vi "SEC code V4.9.vi"() -> ()   [LabVIEW 2022 SP3]
uses:
  SEC code V3.1/Drivers and Aux files/user.lib/atmcd32d.llb/Shutter_type typedef.ctl
  C:/SEC Software V4.91/EcoChemie.Autolab.Sdk.dll
  EcoChemie.Autolab.Sdk.dll
  SEC code V3.1/Drivers and Aux files/State.ctl
  SEC code V3.1/Drivers and Aux files/SECenumctl.ctl
  SEC code V3.1/Drivers and Aux files/user.lib/atmcd32d.llb/TriggerMode_mode typedef.ctl
  SEC code V3.1/Drivers and Aux files/OSSPEC.ctl
  SEC code V3.1/Drivers and Aux files/OSPEC-enum.ctl
  Labview/IVIUM/IVIUM_remdriver.lvlib
panel:
  out "Current PD 2":dbl
  out "POtential PD 2":dbl
  in  "Tab Control 5":enum32{"AUTOLAB", "IVIUM", "iDUS", "Kymera"}(tab)
  out "current":dbl
  out "Error after autolab connection?":errorcluster
  out "Autolab Connected?":bool
  out "Voltage":dbl format="%#_3e"
  out "PotentialOverload":bool
  out "Bandwidth":i32
  out "CurrentRange":i32
  out "Mode":i32
  out "Measured voltage":dbl
  out "CurrentOverload":bool
  out "Cell on?":bool
  out "current":dbl caption="Current (A)" format="%_4g"
  out "cell on":bool
  out "V (during measurment)":dbl
  out "Potentiostat Status":string
  out "T reached?":bool
  out "Shut down sequence run?":bool
  out "Curent Temp":i32
  in  "Tab Control 4":T1(tab)
  in  "Use autolab?":bool=TRUE
  in  "Embedded Exe File":path=path "C:/Program Files/Metrohm Autolab/Autolab SDK 2.1/Hardware Setup Files/Adk.x"
  in  "Hardware Setup File":path=path "C:/ProgramData/Metrohm Autolab/13.0/HardwareSetup.AUT55157.xml"
  in  "Bandwidth 2":i32(ring)=2 items=["UltraHigh_Speed", "High_Speed", "High_Stability"]
  in  "Start potential (V)":dbl=0.2
  in  "Stop potential (V)":dbl=0.7
  in  "Increment (V)":dbl=0.05
  in  "Default Potential (V)":dbl=0.2
  in  "Wait before \nspectrum (s)":dbl=0.1
  in  "Equilibration \ntime (s)":u32=5
  in  "Reverse Scan\ndirection":bool
  in  "(update and read)":bool
  in  "Tab Control 3":T2(tab)=enum."iDUS run"
  in  "Inetegration\n Time (us)":i32=5000
  in  "Continuous \nStrobe Delay (us)":i32
  in  "Number of averages":i32
  in  "Use iDus?":bool=TRUE
  in  "Return detector \nto room T?":bool
  in  "Init, Cool, read dark,\nOR\nWarm/de-init detector":bool
  in  "Temperature\n(degrees C)":i32=-80
  in  "Number of scans in kinetic cycle":i32=30
  in  "Exposure time (s)":dbl=0.03
  in  "Tab Control 2":T3(tab)
  in  "V 1 time (s)":dbl=10.0
  in  "V off time":dbl=30.0
  in  "Sampling\n delay (s)":dbl
  in  "V 2 time (s)":dbl=20.0
  in  "Run OSPSEC":bool
  in  "Square wave?":bool
  out "OCP I (close to 0)":dbl
  out "OCP":dbl format="%_3f"
  in  "V1 (V)":dbl=0.4
  in  "V2 (V)":dbl=0.8
  in  "Slow sample time (s)":dbl=1500.0
  out "Time during PD":u32
  in  "File Name":string="test-1"
  in  "File Path":path=path "C:/Data"
  in  "Tab Control":T4(tab)
  out "?":T5(graph)
  out "?":cluster{i32[], dbl[]}(graph)
  out "?":T5(graph)
  out "?":T5(graph)
  out "Current during PD":dbl(graph)=1.602783203125e-06
  out "?":cluster{dbl[], dbl[]}(graph)
  out "Potential  During PD":dbl(graph)=-0.0002471923828124972
  out "Setpoint":dbl
  out "?":cluster{i32[], "array":i32[]}(graph)
  out "I_overload":bool
  out "Aninput1_overload":bool
  out "E_overload":bool
  out "cell-off button pressed":bool
  in  "Default\nCurrent range":T6(ring)=enum."100 uA"
  in  "Default Filter":T7(ring)=enum."10 kHz"
  out "Device serial number":string
  in  "Set Stability":T8(ring)=enum."Standard"
  out "Number of Spectrometers":i32
  out "IDus not in read loop? (kinetic)":bool
  out "Get status return code":dbl
  out "xpixels":i32
  out "ypixels":i32
  out "Calculated exposure time":sgl format="%.2f"
  out "Check timings return code":u32
  out "Set temprature\nreturn code":u32
  out "get aquired data return code":u32
  out "Start Aquisition return code":u32
  out "Init. return code":u32
  out "Cooler Off return code":u32
  out "Time before the start of current aquisition (ms)":u32
  out "Time  after the aquisition (before fetch data), (ms)":u32
  in  "Shutter opens on TTL":T9=enum."TTL High"
  in  "Shutter open and close time":i32
  out "Get aqisition ok? (kinetic mode)":bool
  out "Time taken to apply V2":u32
  out "Values to re-intialise to at end\nof the measument":T10
  out "V2 applied?":bool
  out "ContinuousStrobe Out":u32
  out "Wrapper Out":u32
  out "WL Values":dbl[](array[numeric])
  out "Number of time the OCEAN averaging loop has run -1":i32
  out "Adc":refnum<k24>
  out "Sampler 2":refnum<k24>
  out "Dio":refnum<k24>
  out "Dac":refnum<k24>
  out "instrument":refnum<k24>
  out "Ei":refnum<k24>
  out "AutolabConnection":refnum<k24>
  out "EI status supported for":string[](array[string])
  out "TemperatureOverload":bool
  out "ManualCellSwitch":bool
  out "Oscillation":bool
  out "PD ENDED\nEXIT MEASURMENT":bool=TRUE
  out "Current PD":dbl
  out "POtential PD":dbl
  in  "Exit and disconnect":bool
  # "Program control"
  # "Potential decay control"
  # "Spectrometer control"
  # "System status"
  # "SEC control"
  # "Cell on?"
  # "Use the integration time program in the same folder as this program\nto get the optimum value. For kinetic mode the time resolution is limited \nby integration time"
  # "Unless you know what you are doing keep these at 0.03 and 30"
  # "I overload overload"
  # "off button pressed"
  # "Aninput1 overload"
  # "E overload"
  # "OSPEC loop exit"
  # "Checklist for avoiding errors:\n(1) Light on the IVIUM should be blue with red flashes\nIf the system crahes and the light is red then connect and disconnect in IVUM soft/turn stat off/on\n(2) Maya Pro should read in ocean view/or the get intensity program\nIf maya is not reading connect and disconnect USB.\n(3) If errors persist rrepeat steps 1 + 2 then re-compile code by clicking the\nwhite (run) whilst holding down CRTL + (left) SHIFT\n(4) IF USING THE iDus DO NOT EXIT WITHOUT WARMING CAMERA BACK TO ROOM T,YOU \nWILL DAMAGE IT \n(6) if the IVIUM.dll does not load click broken arrows and \"show error\" until you see the call library function (see blue circles). Double click on this and paste the following into the directory (red circle):   \n%windir%\\Labview\\IVIUM\\IVIUM_remdriver.dll"
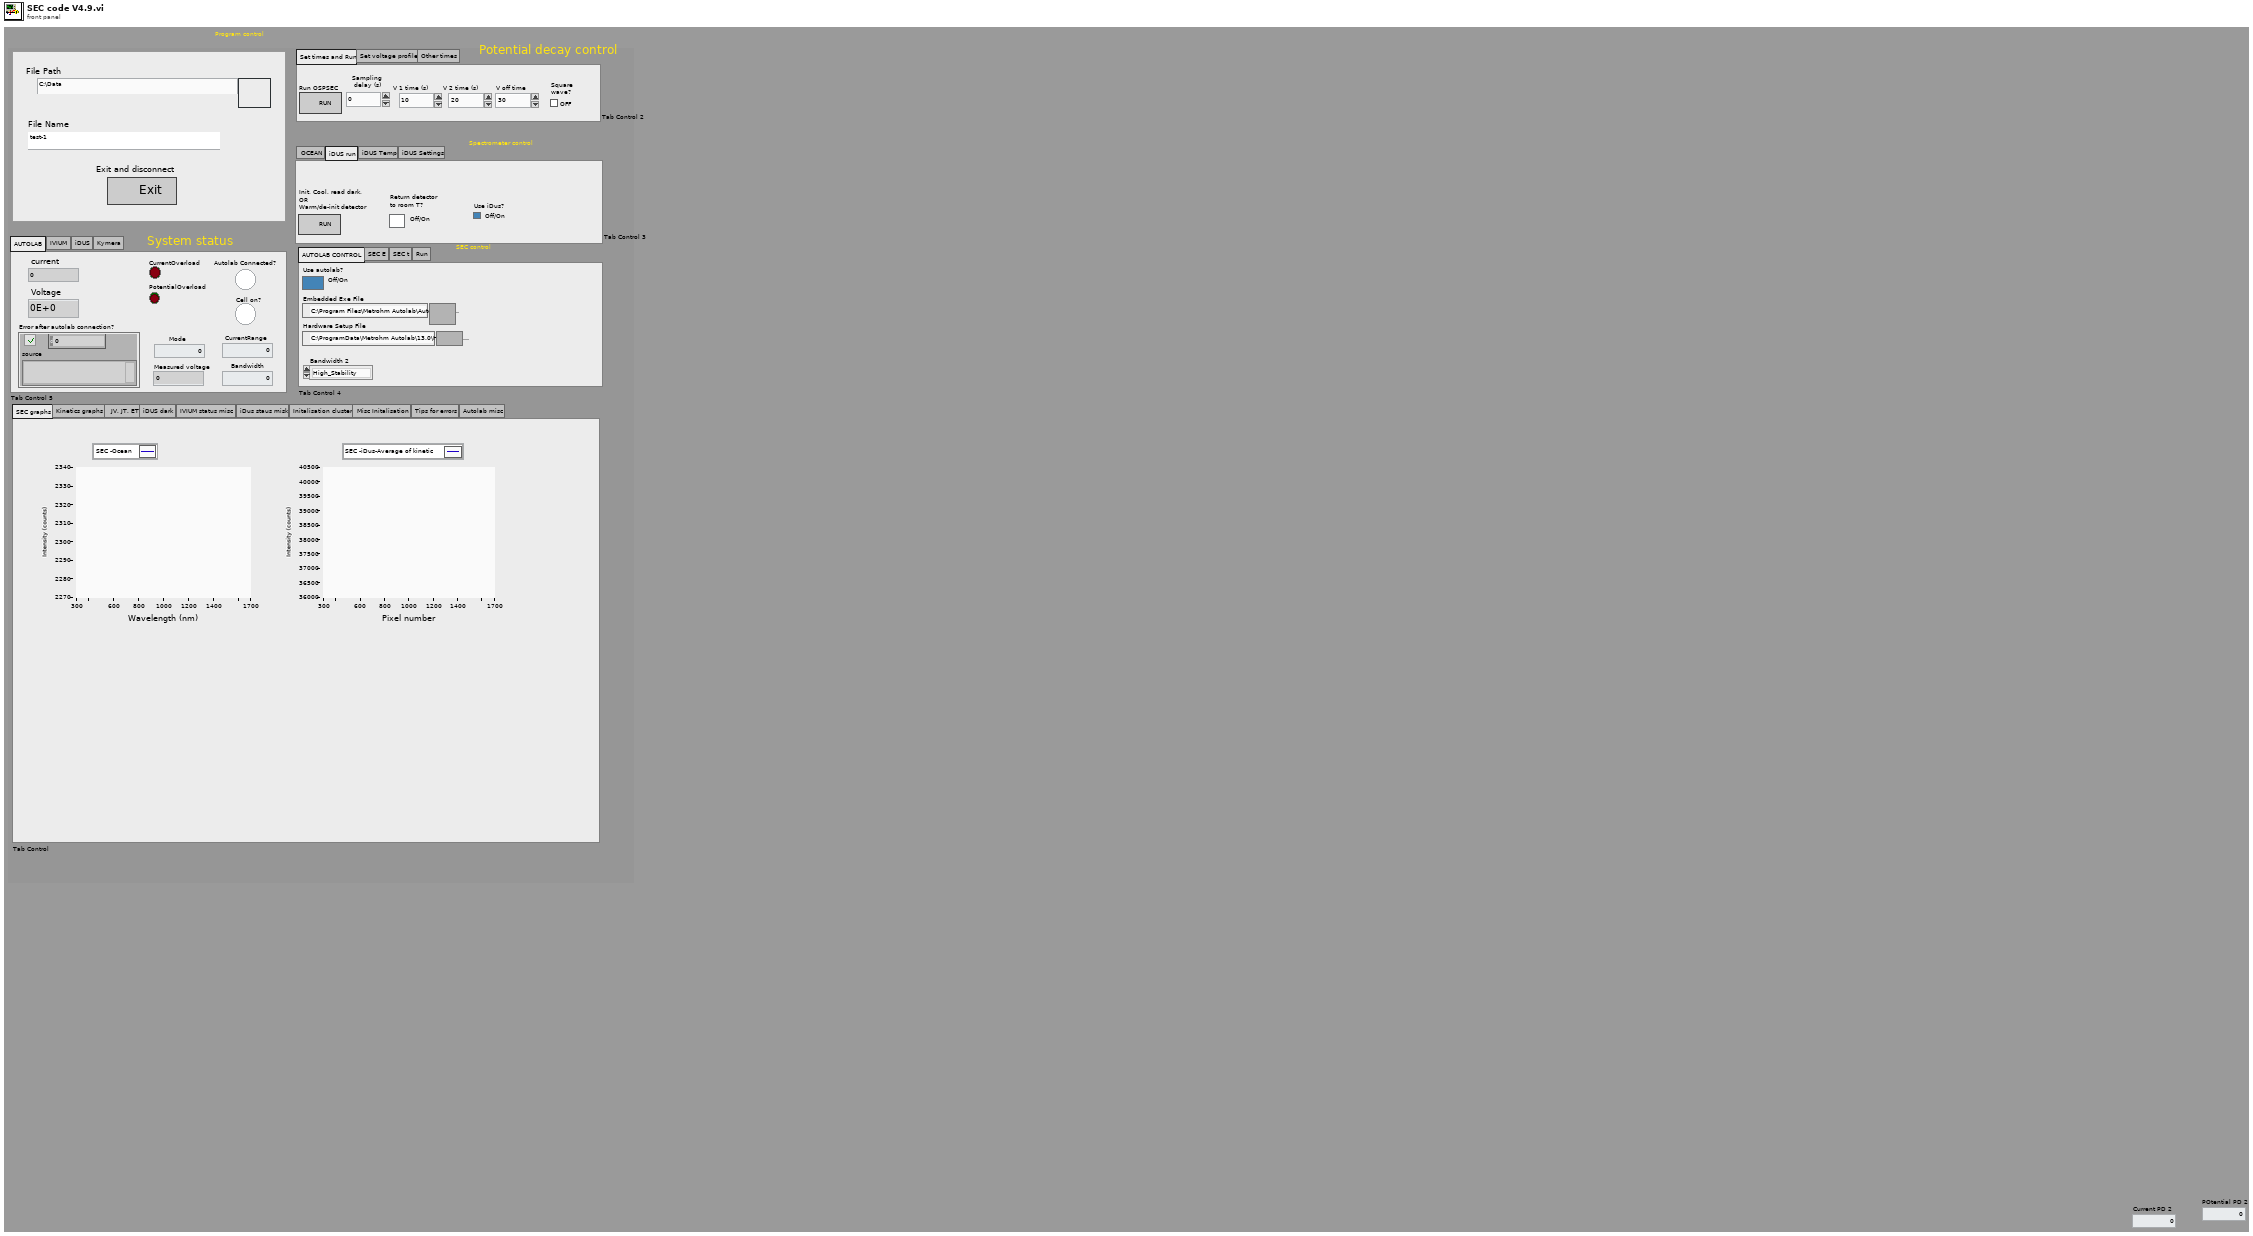
[diagram p1: front panel]
types:
  T1 = enum32{"AUTOLAB CONTROL", "SEC E", "SEC t", "Run"}
  T2 = enum32{"OCEAN", "iDUS run", "iDUS Temp", "iDUS Settings"}
  T3 = enum32{"Set times and Run", "Set voltage profile", "Other times"}
  T4 = enum32{"SEC graphs", "Kinetics graphs", " JV, JT, ET", "iDUS dark", "IVIUM status misc", "iDus staus misk", "Initalisation cluster", "Misc Initalisation ", "Tips for errors", "Autolab misc"}
  T5 = cluster{"WL Values":dbl[], "Spectrum Values":dbl[]}
  T6 = enum16{"10 A", "1 A", "100 mA", "10 mA", "1 mA", "100 uA", "10 uA", "1 uA", "100 nA", "10 nA", "1 nA", "100 pA", "10 pA", "1 pA"}
  T7 = enum16{"1 MHz", "100 kHz", "10 kHz", "1 kHz", "10 Hz"}
  T8 = enum16{"High Speed", "Standard", "High Stability"}
  T9 = typedef "Shutter_type typedef.ctl" = enum16{"TTL Low", "TTL High"}
  T10 = cluster{"Currents":dbl[], "Potentials":dbl[], "Device Status":string, "Device serial no":string, "Current":dbl, "Default \nPotential":dbl, "I overload":bool, "Cell On":bool, "E overload":bool, "Aninput1 overload":bool, "Cell off button pressed":bool, "Start potential":dbl, "Stop potential":dbl, "Increment":dbl, "SEC":dbl[], "Path":path, "File name":string}
  T11 = cluster{"Current array":dbl[], "Potential array":dbl[], "Status":string, "Serial No":string, "Current":dbl, "Default\n potential":dbl, "I overload":bool, "Cell on":bool, "E overload":bool, "Cell of button pressed":bool, "Aninput1 overload":bool, "Stop \npotential":dbl, "Start \npotential":dbl, "Increment":dbl, "Spectrum":dbl[][], "Path":path, "File Name":string, "Sample rate":dbl, "V2 time":dbl, "V off time":dbl, "V 2":dbl, "V 1":dbl, "V1 time":dbl, "Time array":dbl[], "Integration time":i32, "Continous strobe delay":i32, "Time elapsed ":i32, "Start time":i32, "Time for E measurment":i32[], "Time for I measurment ":i32[], "Time for spectrum measurment":i32[], "Return detector to \nroom T":bool, "Number of scans in kinetic cycle":i32, "Exposure time":dbl}
  T12 = typedef "State.ctl" = enum16{"Initialize", "Wait for Event", "Run SEC", "Run OSPEC", "Initialse and cool iDus", "Exit"}
  T13 = typedef "SECenumctl.ctl" = enum16{"Read spectrum from Ocean", "Read spectrum from iDus", "Apply potential", "Wait", "Apply potential Autolab"}
  T14 = typedef "TriggerMode_mode typedef.ctl" = enum16{"Internal", "External", "N/A (2)", "N/A (3)", "N/A (4)", "N/A (5)", "External Start", "External Exposure (Bulb)", "N/A (8)", "External FVB EM", "Software", "N/A (11)", "External Charge Shifting"}
  T15 = typedef "OSSPEC.ctl" = enum16{"Read Potential and spectrum", "Read current and spectrum", "Reinitialise Cell", "Apply V1", "End measurment", "Apply V2"}
  T16 = typedef "OSPEC-enum.ctl" = enum16{"Check exit", "Read", "Wait"}
  T17 = enum16{"off", "EStat4EL", "EStat2EL", "EStatDummy1", "EStatDummy2", "EStatDummy3", "EStatDummy4", "IStat4EL", "IStat2EL", "IStatDummy", "BiStat4EL", "BiStat2EL"}
  T18 = cluster{"Current array":dbl[], "Potential array":dbl[], "Status":string, "Serial No":string, "Current":dbl, "Default\n potential":dbl, "I overload":bool, "Cell on":bool, "E overload":bool, "Cell of button pressed":bool, "Aninput1 overload":bool, "Stop \npotential":dbl, "Start \npotential":dbl, "Increment":dbl, "Spectrum":dbl[][], "Path":path, "File Name":string, "Sample rate":dbl, "V2 time":dbl, "V off time":dbl, "V 2":dbl, "V 1":dbl, "V1 time":dbl, "Time array":dbl[], "Integration time":i32, "Continous strobe delay":i32, "Time elapsed ":i32, "Start time":i32, "Time for E measurment":i32[], "Time for I measurment ":i32[], "Time for spectrum measurment":i32[], "Return detector to \nroom T":bool, "Number of scans in kinetic cycle":i32, "Exposure time":i32}
  T19 = typedef "Error Code Enum typedef.ctl" = enum32{"N/A (0)", "DRV_ERROR_CODES", "DRV_SUCCESS", "DRV_VXDNOTINSTALLED", "DRV_ERROR_SCAN", "DRV_ERROR_CHECK_SUM", "DRV_ERROR_FILELOAD", "DRV_UNKNOWN_FUNC", "DRV_ERROR_VXD_INIT", "DRV_ERROR_ADDRESS", "DRV_ERROR_PAGELOCK", "DRV_ERROR_PAGEUNLOCK", "DRV_ERROR_BOARDTEST", "DRV_ERROR_ACK", "DRV_ERROR_UP_FIFO", "DRV_ERROR_PATTERN", "N/A (16)", "DRV_ACQUISITION_ERRORS", "DRV_ACQ_BUFFER", "DRV_ACQ_DOWNFIFO_FULL", "DRV_PROC_UNKONWN_INSTRUCTION", "DRV_ILLEGAL_OP_CODE", "DRV_KINETIC_TIME_NOT_MET", "DRV_ACCUM_TIME_NOT_MET", "DRV_NO_NEW_DATA", "N/A (25)", "DRV_SPOOLERROR", "N/A (27)", "N/A (28)", "N/A (29)", "N/A (30)", "N/A (31)", "N/A (32)", "DRV_TEMPERATURE_CODES", "DRV_TEMPERATURE_OFF", "DRV_TEMPERATURE_NOT_STABILIZED", "DRV_TEMPERATURE_STABILIZED", "DRV_TEMPERATURE_NOT_REACHED", "DRV_TEMPERATURE_OUT_RANGE", "DRV_TEMPERATURE_NOT_SUPPORTED", "DRV_TEMPERATURE_DRIFT", "N/A (41)", "N/A (42)", "N/A (43)", "N/A (44)", "N/A (45)", "N/A (46)", "N/A (47)", "N/A (48)", "DRV_GENERAL_ERRORS", "DRV_INVALID_AUX", "DRV_COF_NOTLOADED", "DRV_FPGAPROG", "DRV_FLEXERROR", "DRV_GPIBERROR", "N/A (55)", "N/A (56)", "N/A (57)", "N/A (58)", "N/A (59)", "N/A (60)", "N/A (61)", "N/A (62)", "N/A (63)", "DRV_DATATYPE", "DRV_DRIVER_ERRORS", "DRV_P1INVALID", "DRV_P2INVALID", "DRV_P3INVALID", "DRV_P4INVALID", "DRV_INIERROR", "DRV_COFERROR", "DRV_ACQUIRING", "DRV_IDLE", "DRV_TEMPCYCLE", "DRV_NOT_INITIALIZED", "DRV_P5INVALID", "DRV_P6INVALID", "DRV_INVALID_MODE", "DRV_INVALID_FILTER", "DRV_I2CERRORS", "DRV_I2CDEVNOTFOUND", "DRV_I2CTIMEOUT", "DRV_P7INVALID", "N/A (84)", "N/A (85)", "N/A (86)", "N/A (87)", "N/A (88)", "N/A (89)", "DRV_IOCERROR", "DRV_VRMVERSIONERROR"}
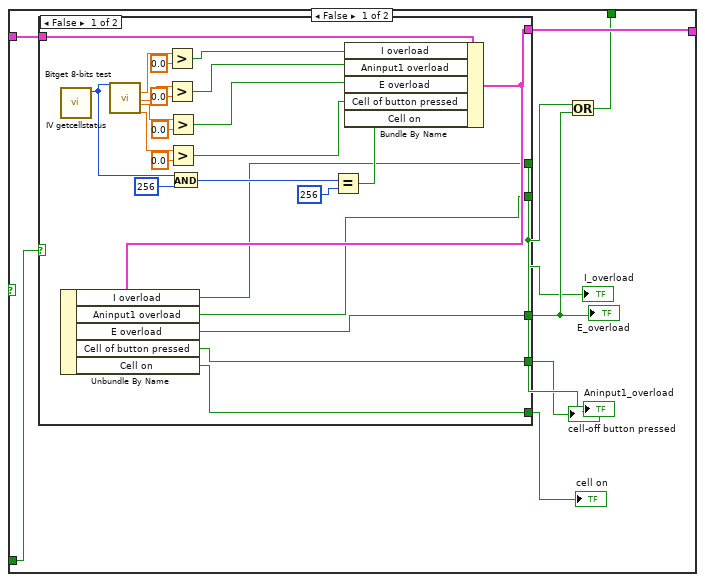
[diagram p2: hidden frame]
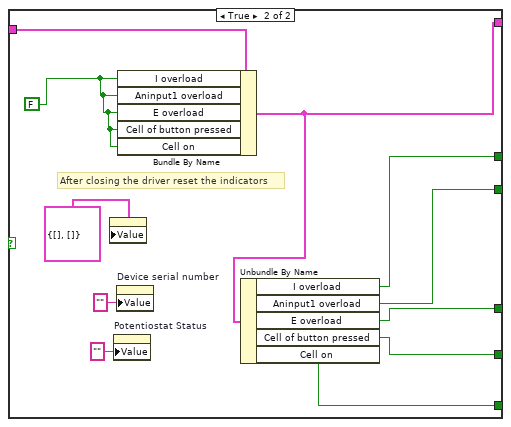
[diagram p3: hidden frame]
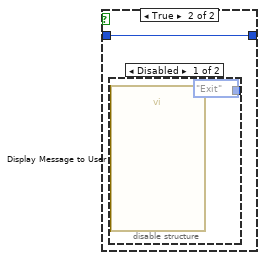
[diagram p4: hidden frame]
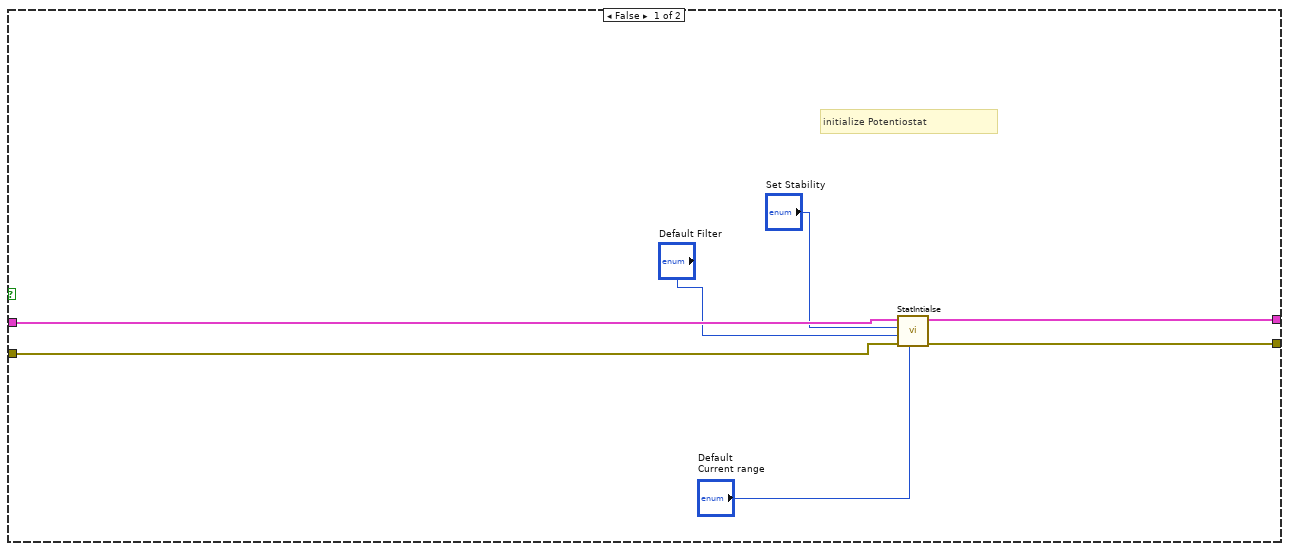
[diagram p7: hidden frame]
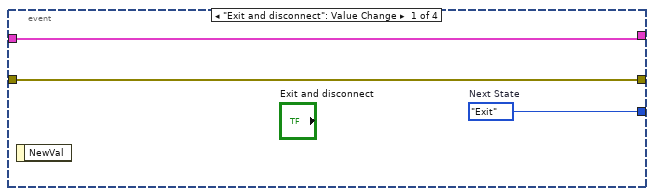
[diagram p9: hidden frame]
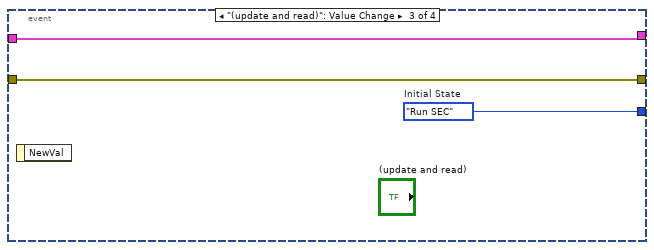
[diagram p10: hidden frame]
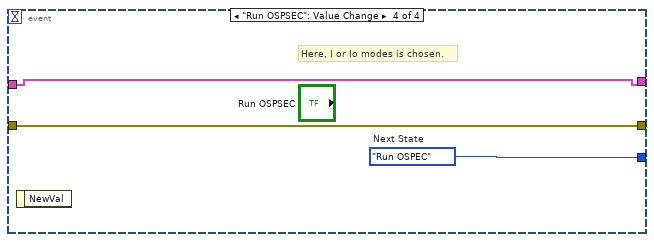
[diagram p11: hidden frame]
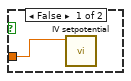
[diagram p12: hidden frame]
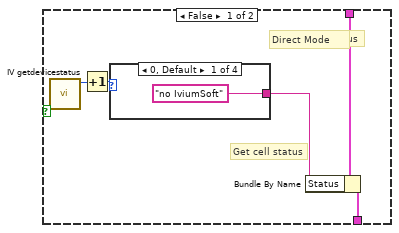
[diagram p13: hidden frame]
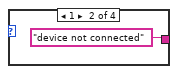
[diagram p14: hidden frame]
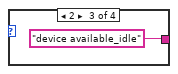
[diagram p15: hidden frame]
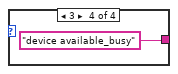
[diagram p16: hidden frame]
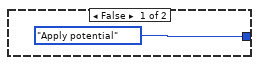
[diagram p17: hidden frame]
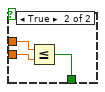
[diagram p20: hidden frame]
diagram:
  w1 = T11 {"Current array"=[], "Potential array"=[], "Status"="", "Serial No"="", "Current"=0.0, "Default\n potential"=0.0, "I overload"=FALSE, "Cell on"=FALSE, "E overload"=FALSE, "Cell of button pressed"=FALSE, "Aninput1 overload"=FALSE, "Stop \npotential"=0.0, "Start \npotential"=0.0, "Increment"=0.0, "Spectrum"=[], "Path"=path "", "File Name"="", "Sample rate"=0.0, "V2 time"=0.0, "V off time"=0.0, "V 2"=0.0, "V 1"=0.0, "V1 time"=0.0, "Time array"=[], "Integration time"=0, "Continous strobe delay"=0, "Time elapsed "=0, "Start time"=0, "Time for E measurment"=[], "Time for I measurment "=[], "Time for spectrum measurment"=[], "Return detector to \nroom T"=FALSE, "Number of scans in kinetic cycle"=0, "Exposure time"=0.0}  # Init cluster
  w3 = State."Initialize"  # Initial State
  n1 = while {
    shift-right: [w21] -> _
    shift-left: w3 -> [w38]
    shift-right: [w24] -> _
    shift-left: w1 -> [w17]
    shift-right: [w25] -> _
    shift-left: errorcluster {"status"=FALSE, "code"=0, "source"=""} ("error constant") -> [w37]
    stop <- w35 stop-if-true
    # "Main VI State Machine"
    n2 = Bundle By Name(cluster=w17, "Sample rate"="Sampling\n delay (s)", "V1 time"="V 1 time (s)", "V2 time"="V 2 time (s)", "V off time"="V off time", "V 2"="V2 (V)", "V 1"="V1 (V)", "Integration time"="Inetegration\n Time (us)", "Continous strobe delay"="Continuous \nStrobe Delay (us)", "Exposure time"="Exposure time (s)", "Number of scans in kinetic cycle"="Number of scans in kinetic cycle") -> (w11:T11)
    n3 = Bundle By Name(cluster=w11, "Default\n potential"="Default Potential (V)", "Start \npotential"="Start potential (V)", "Stop \npotential"="Stop potential (V)", "Increment"="Increment (V)", "Path"="File Path", "File Name"="File Name") -> (w23:T11)
    n4 = case shown="\"Run SEC\"" w38 {
      tunnel: [w94 w137 w185 w504 w544 w1716] -> w7
      tunnel: [w93 w134 FALSE ("Stop Loop?") w501 FALSE ("Stop Loop?") _] -> w36
      tunnel: w23 -> [w91 w131 w174 w505 w543 w1714]
      tunnel: [w90 w132 w159 w505 w539 w1714] -> w31
      tunnel: w37 -> [w95 w136 w183 w507 w541 w1713]
      tunnel: [w96 w135 w182 w508 w540 w1713] -> w25
      tunnel: [1 ("devconnect") 1 ("devconnect") 1 ("devconnect") w506 1 ("devconnect") 1 ("devconnect")] -> w22
      frame "Initialize" {
        w93 = FALSE  # Stop Loop?
        w94 = State."Wait for Event"  # Next State
        # "Initialize - Initialize variables needed"
        n5 = case shown="True" "Use autolab?" {
          tunnel: [w104 w109] -> w96
          tunnel: w95 -> [w103 _]
          tunnel: w91 -> [w102 w111]
          tunnel: [w98 w111] -> w90
          frame False {
            # "initialize Potentiostat"
            n6 = call "StatIntialse.vi"("Init cluster 2"=w102, "Set Stability"="Set Stability", "Default\n Filter"="Default Filter", "error in (no error)"=w103, "Default\nCurrent range"="Default\nCurrent range") -> ("Init cluster"=w98:T18, "error out"=w104:errorcluster)  [unwired: 4 in]
          }
          frame True {
            w108 = 2 items=["UltraHigh_Speed", "High_Speed", "High_Stability"] ("Bandwidth")
            w113 = 0 items=["Potentiostatic", "Galvanostatic"] ("Mode")
            w114 = -4 items=["CR07_1A"=0, "CR06_10A"=1, "CR01_100A"=2, "CR00_1000A"=3, "CR05_20A"=20, "CR04_40A"=40, "CR03_50A"=60, "CR02_80A"=80, "CR19_1pA"=-12, "CR18_10pA"=-11, "CR17_100pA"=-10, "CR16_1nA"=-9, "CR15_10nA"=-8, "CR14_100nA"=-7, "CR13_1uA"=-6, "CR12_10uA"=-5, "CR11_100uA"=-4, "CR10_1mA"=-3, "CR09_10mA"=-2, "CR08_100mA"=-1] ("CurrentRange")
            w115 = 1 items=["Off", "On"] ("CellOnOff")
            n7 = call "Connect AutoLab.vi"("Embedded Exe File"="Embedded Exe File", "Hardware Setup File"="Hardware Setup File") -> ("error out"=w120:errorcluster, ".NET Refnum out"=w129:refnum<k24>)  [unwired: 8 in]
            "Error after autolab connection?" <- w120
            n8 = property class="Instrument"(reference=w129, error in=w120) -> (reference out=→"instrument":refnum<k24>, error out=w121:errorcluster, "Adc"=→"Adc":refnum<k24>, "Dac"=→"Dac":refnum<k24>, "Dio"=→"Dio":refnum<k24>, "AutolabConnection"=w117:refnum<k24>, "Ei"=w107:refnum<k24>)
            "AutolabConnection" <- w117
            n9 = property class="AutolabConnection"(reference=w117) -> ("IsConnected"=→"Autolab Connected?":bool)  [unwired: 1 in, 2 out]
            n10 = property class="EI"(reference=w107, error in=w121) -> (reference out=→"Ei":refnum<k24>, error out=w128:errorcluster, "Sampler"=→"Sampler 2":refnum<k24>)
            n11 = Unbundle By Name(w111) -> ("Default\n potential"=w110:dbl)
            n12 = Build Array(w121, w128) -> (w122:errorcluster[])
            n13 = Merge Errors(w122) -> (w112:errorcluster)
            n14 = property class="EI" props=["Bandwidth", "CellOnOff", "CurrentRange", "Mode", "Setpoint", "Current", "Potential", "PotentialApplied", "PotentialOverload", "Sampler", "Setpoint", "PotentialOverload"](reference=w107, error in=w112, "Bandwidth"=w108, "CellOnOff"=w115, "CurrentRange"=w114, "Mode"=w113, "Setpoint"=w110) -> (error out=w109:errorcluster)  [unwired: 8 out]
            n15 = property class="EI"(reference=w107) -> ("Potential"=w106:dbl, "Current"=w105:dbl)  [unwired: 1 in, 2 out]
            n16 = property on="current" class="DigNum (strict)"("Value"=w105) -> ()  [unwired: 2 in, 2 out]
            n17 = property on="Voltage" class="DigNum (strict)"("Value"=w106) -> ()  [unwired: 2 in, 2 out]
          }
        }
        n18 = property on="V2 applied?" class="Bool (strict)"("Value"=FALSE ("V2 applied")) -> ()  [unwired: 2 in, 2 out]
        "Values to re-intialise to at end\nof the measument" <- T10 {"Currents"=[], "Potentials"=[], "Device Status"="", "Device serial no"="", "Current"=0.0, "Default \nPotential"=0.0, "I overload"=FALSE, "Cell On"=FALSE, "E overload"=FALSE, "Aninput1 overload"=FALSE, "Cell off button pressed"=FALSE, "Start potential"=0.0, "Stop potential"=0.0, "Increment"=0.0, "SEC"=[], "Path"=path "", "File name"=""} ("Values to re-intialise to at end\nof the measument")
      }
      frame "Wait for Event" {
        w134 = FALSE  # Stop Loop?
        # "Wait for Event - Use an Event Structure to monitor the user interface for events that run different states of the state machine."
        n19 = event shown="[1] \"Init, Cool, read dark, OR Warm/de-init detector\": Value Change" {
          selector: _ -> [_ _ _ _]
          dyn-events: _ -> [_ _ _ _]
          timeout: _ -> [_ _ _ _]
          tunnel: [w140 State."Initialse and cool iDus" ("Next State") w147 w151] -> w137
          tunnel: w136 -> [w139 w145 w148 w150]
          tunnel: [w139 w145 w148 w150] -> w135
          tunnel: w131 -> [w138 w143 w146 w149]
          tunnel: [w138 w141 w146 w149] -> w132
          event "Exit and disconnect": Value Change {
            w140 = State."Exit"  # Next State
            n20 = event-data() -> ()  [unwired: 1 in, 1 out]
          }
          event "Init, Cool, read dark,\nOR\nWarm/de-init detector": Value Change {
            n21 = event-data() -> ()  [unwired: 1 in, 4 out]
            n22 = Bundle By Name(cluster=w143, "Return detector to \nroom T"="Return detector \nto room T?") -> (w141:T11)
          }
          event "(update and read)": Value Change {
            w147 = State."Run SEC"  # Initial State
            n23 = event-data() -> ()  [unwired: 1 in, 1 out]
          }
          event "Run OSPSEC": Value Change {
            w151 = State."Run OSPEC"  # Next State
            # "Here, I or Io modes is chosen."
            n24 = event-data() -> ()  [unwired: 1 in, 1 out]
          }
        }
      }
      frame "Run SEC" {
        w185 = State."Wait for Event"  # Next State
        n25 = property on="Use autolab?" class="Bool (strict)"() -> ("Value"=w154:bool)  [unwired: 2 in, 2 out]
        n26 = case shown="True" w154 {
          tunnel: w174 -> [w191 w199]
          tunnel: [w190 w199] -> w161
          frame False {
            # "Get cell status"
            # "Get Device Status"
            # "Direct Mode"
            n27 = call "IV getdevicestatus.vi"() -> ("return type"=w193:i32)  [unwired: 10 in, 1 out]
            n28 = Increment(x=w193) -> (x+1=w192:i32)
            n29 = case shown="0, Default" w192 {
              tunnel: ["no IviumSoft" "device not connected" "device available_idle" "device available_busy"] -> w194
              frame 0, Default {
              }
              frame 1 {
              }
              frame 2 {
              }
              frame 3 {
              }
            }
            n30 = Bundle By Name(cluster=w191, "Status"=w194) -> (w190:T11)
          }
          frame True {
          }
        }
        n31 = property on="Use autolab?" class="Bool (strict)"() -> ("Value"=w156:bool)  [unwired: 2 in, 2 out]
        n32 = case shown="True" w156 {
          tunnel: [SECenumctl."Apply potential" SECenumctl."Apply potential Autolab"] -> w181
          frame False {
          }
          frame True {
          }
        }
        n33 = Unbundle By Name(w161) -> ("Increment"=w180:dbl, "Start \npotential"=w184:dbl, "Stop \npotential"=w175:dbl)
        n34 = while {
          shift-right: [w227] -> w158
          shift-left: w161 -> [w228]
          tunnel: w180 -> [w223]
          tunnel: w184 -> [w222]
          shift-right: [w224] -> w182
          shift-left: w183 -> [w225]
          shift-right: [w216] -> _
          shift-left: w181 -> [w220]
          shift-right: [w218] -> w160
          shift-left: dbl[] [0.0] -> [w217]
          shift-right: [w213] -> w164
          shift-left: dbl[] [0.0] -> [w214]
          tunnel: w175 -> [w215]
          shift-right: [w212] -> w173
          shift-left: dbl[][] [] -> [w211]
          tunnel: "Reverse Scan\ndirection" -> [w210]
          tunnel: [w208] -> _
          tunnel: [w208] -> _
          shift-right: [w207] -> _
          shift-left: -3 ("y") -> [w206]
          i -> [w226]
          stop <- w208 stop-if-true
          n35 = case shown="\"Apply potential Autolab\"" w220 {
            tunnel: w228 -> [w251 w315 w350 w365 w463]
            tunnel: [w250 w314 w350 w365 w463] -> w227
            tunnel: w226 -> [w264 w324 _ w372 w471]
            tunnel: w225 -> [w261 w306 w346 w374 w472]
            tunnel: [w252 w295 w346 w374 w472] -> w224
            tunnel: w223 -> [w247 w312 _ _ _]
            tunnel: w222 -> [w263 w323 _ _ _]
            tunnel: [w244 w307 w349 w378 w477] -> w221
            tunnel: [w236 w310 w348 w377 w476] -> w219
            tunnel: [w255 w318 w347 w379 w475] -> w218
            tunnel: w217 -> [w256 w319 w347 w379 w475]
            tunnel: [SECenumctl."Wait" SECenumctl."Wait" w351 w360 w459] -> w216
            tunnel: w215 -> [w236 w310 _ _ _]
            tunnel: w214 -> [w254 w317 w342 w380 w473]
            tunnel: [w253 w316 w342 w380 w473] -> w213
            tunnel: [w248 w313 w341 w368 w466] -> w212
            tunnel: w211 -> [w248 w313 w341 w369 w465]
            tunnel: w210 -> [w237 w311 w340 w376 w464]
            tunnel: [w237 w311 w339 w375 w464] -> w209
            tunnel: w206 -> [w235 w305 w337 w362 w460]
            tunnel: [w235 w304 w337 w362 w460] -> w207
            frame "Apply potential", Default {
              # "Here, the while loop iterates three times for every one change of potential. The loop counter is therefore diveded by three, multipled by the increment and then added to the start  potential to give the next potential in the LSV. Potential is applied, then current is read. These go into a build array function . A wait is inclided to alow the sample to equilibriate at the start potential"
              n36 = Divide(x=w264, y=3) -> (x/y=w259:dbl)
              n37 = Multiply(x=w247, y=w259) -> (x*y=w262:dbl)
              n38 = Add(x=w262, y=w263) -> (x+y=w244:dbl)
              "V (during measurment)" <- w244
              n39 = call "IV setpotential.vi"("error in (no error)"=w261, "value"=w244) -> ("error out"=w258:errorcluster)  [unwired: 7 in, 2 out]
              n40 = Equal To 0?(x=w259) -> (x = 0?=w260:bool)
              n41 = case shown="True" w260 {
                tunnel: w258 -> [w274 w276]
                tunnel: [w274 w276] -> w257
                frame False {
                }
                frame True {
                  n42 = Multiply(x=u32 1000, y="Equilibration \ntime (s)") -> (x*y=w275:u32)
                  n43 = Wait (ms)(milliseconds to wait=w275) -> ()  [unwired: 1 out]
                }
              }
              n44 = Equal To 0?(x=w247) -> (x = 0?=w242:bool)
              n45 = Absolute Value(x=w244) -> (abs(x)=w245:dbl)
              n46 = Build Array (concatenate)(w244, w256) -> (w255:dbl[])
              n47 = Greater?(x=w245, y=3.0) -> (0:w243:bool)
              n48 = call "IV getcurrent.vi"("error in (no error)"=w257) -> ("error out"=w240:errorcluster, "value out"=w238:dbl)  [unwired: 8 in, 1 out]
              n49 = Or(x=w242, y=w243) -> (x .or. y?=w241:bool)
              n50 = flat-sequence {
                tunnel: w240 -> [w268]
                tunnel: [w268] -> w239
                tunnel: w238 -> [w267]
                frame #0 {
                  n51 = call "Current ranging routine (SubVI).vi"("Current"=w267) -> ()  [unwired: 11 in]
                  n52 = Wait (ms)(milliseconds to wait=u32 100) -> ()  [unwired: 1 out]
                }
              }
              n53 = case shown="True" w241 {
                frame False {
                }
                frame True {
                  # "abort if E >3 V or\ndelta E =0"
                  n54 = call "IV setcellon.vi"("cellon"=0) -> ("error out"=w272:errorcluster)  [unwired: 8 in, 2 out]
                  n55 = call "IV close.vi"("error in (no error)"=w272) -> ("error out"=w270:errorcluster)  [unwired: 9 in, 1 out]
                  n56 = call "Display Message to User2"("error in (no error)"=w270) -> ("OK"=w273:bool)  [unwired: 9 in, 1 out]
                  n57 = Stop(stop? (T)=w273) -> ()
                }
              }
              n58 = call "IV getcurrent.vi"("error in (no error)"=w239) -> ("error out"=w252:errorcluster, "value out"=w249:dbl)  [unwired: 8 in, 1 out]
              n59 = Bundle By Name(cluster=w251, "Current"=w249) -> (w250:T11)
              n60 = property on="current" class="DigNum (strict)"("Value"=w249) -> ()  [unwired: 2 in, 2 out]
              n61 = Build Array (concatenate)(w249, w254) -> (w253:dbl[])
            }
            frame "Apply potential Autolab" {
              w308 = 1 items=["Off", "On"] ("CellOnOff")
              w303 = 0 items=["Potentiostatic", "Galvanostatic"] ("Mode")
              # "Here, the while loop iterates three times for every one change of potential. The loop counter is therefore diveded by three, multipled by the increment and then added to the start  potential to give the next potential in the LSV. Potential is applied, then current is read. These go into a build array function . A wait is inclided to alow the sample to equilibriate at the start potential"
              n62 = Divide(x=w324, y=3) -> (x/y=w320:dbl)
              n63 = Multiply(x=w312, y=w320) -> (x*y=w322:dbl)
              n64 = Add(x=w322, y=w323) -> (x+y=w307:dbl)
              "Voltage" <- w307
              n65 = property on="Ei" class="Ref (strict)"() -> ("Value"=w282:refnum<k24>)  [unwired: 2 in, 2 out]
              n66 = property class="EI"(reference=w282, error in=w306, "Bandwidth"="Bandwidth 2", "CellOnOff"=w308, "CurrentRange"=w305, "Mode"=w303, "Setpoint"=w307) -> (error out=w287:errorcluster)  [unwired: 1 out]
              n67 = Equal To 0?(x=w320) -> (x = 0?=w321:bool)
              n68 = case shown="True" w321 {
                tunnel: w287 -> [w332 w335]
                tunnel: [w332 w335] -> w299
                frame False {
                }
                frame True {
                  n69 = property on="Equilibration \ntime (s)" class="DigNum (strict)"() -> ("Value"=w333:u32)  [unwired: 2 in, 2 out]
                  n70 = Multiply(x=u32 1000, y=w333) -> (x*y=w334:u32)
                  n71 = Wait (ms)(milliseconds to wait=w334) -> ()  [unwired: 1 out]
                }
              }
              n72 = property on="Sampler 2" class="Ref (strict)"() -> ("Value"=w280:refnum<k24>)  [unwired: 2 in, 2 out]
              n73 = property class="EI"(reference=w282, error in=w287) -> (error out=w286:errorcluster, "EiStatusSupportedFor"=→"EI status supported for":string[])  [unwired: 1 out]
              n74 = invoke class="Sampler" method="Sample"(reference=w280, error in=w287) -> (error out=w285:errorcluster)  [unwired: 1 in, 2 out]
              n75 = Build Array (concatenate)(w307, w319) -> (w318:dbl[])
              n76 = property class="EI"(reference=w282, error in=w299) -> (reference out=w281:refnum<k24>, error out=w298:errorcluster, "Bandwidth"=→"Bandwidth":i32, "CurrentRange"=→"CurrentRange":i32, "Mode"=→"Mode":i32, "Setpoint"=w296:dbl, "Current"=w297:dbl)
              "Measured voltage" <- w296
              n77 = flat-sequence {
                tunnel: w298 -> [w330]
                tunnel: [w330] -> w284
                tunnel: [w329] -> w304
                tunnel: w297 -> [w328]
                tunnel: w296 -> [w327]
                frame #0 {
                  n78 = Wait (ms)(milliseconds to wait=u32 100) -> ()  [unwired: 1 out]
                  n79 = call "Range_selector.vi"("potential"=w327, "current"=w328) -> ("range integer"=w329:i32)  [unwired: 9 in]
                }
              }
              n80 = Merge Errors(w284, w286, w285) -> (w283:errorcluster)
              n81 = call "P_Stat_Status1.vi"("error in (no error)"=w283, ".NET Refnum in"=w281) -> ("error out"=w289:errorcluster, "ManualCellSwitch"=→"ManualCellSwitch":bool, "Oscillation"=→"Oscillation":bool, "TemperatureOverload"=→"TemperatureOverload":bool, "CurrentOverload"=→"CurrentOverload":bool, "Cell"=→"Cell on?":bool)  [unwired: 3 in, 1 out]
              n82 = property class="EI"(reference=w281, error in=w289) -> (error out=w295:errorcluster, "Current"=w279:dbl)  [unwired: 1 out]
              "current" <- w279
              n83 = Bundle By Name(cluster=w315, "Current"=w279) -> (w314:T11)
              n84 = property on="current" class="DigNum (strict)"("Value"=w279) -> ()  [unwired: 2 in, 2 out]
              n85 = Build Array (concatenate)(w279, w317) -> (w316:dbl[])
            }
            frame "Wait" {
              n86 = Multiply(x="Wait before \nspectrum (s)", y=1000.0) -> (x*y=w345:dbl)
              n87 = Wait (ms)(milliseconds to wait=w345) -> ()  [unwired: 1 out]
              n88 = case shown="False" "Use iDus?" {
                tunnel: [SECenumctl."Read spectrum from Ocean" SECenumctl."Read spectrum from iDus"] -> w351
                frame False {
                }
                frame True {
                }
              }
              n89 = case shown="False" w340 {
                selector: w340 -> [w354 w357]
                tunnel: [0.0 1.0] -> w349
                tunnel: [1.0 ("Stop \npotential") 0.0 ("Stop \npotential")] -> w348
                tunnel: [w354 w357] -> w339
                frame False {
                }
                frame True {
                }
              }
            }
            frame "Read spectrum from iDus" {
              n90 = Unbundle By Name(w365) -> ("Exposure time"=w373:dbl, "Number of scans in kinetic cycle"=w366:i32)
              n91 = Equal?(x=w372, y=2) -> (x = y?=w370:bool)
              n92 = Multiply(x=1024, y=w366) -> (x*y=w383:i32)
              n93 = stacked-sequence {
                seq-local: [_ _ _ _ _ _ _ _ _ _ w416 _] -> [_ _ _ _ _ _ _ _ _ _ _ w425]
                tunnel: [_ _ _ _ _ _ _ _ _ _ _ w426] -> w381
                tunnel: w366 -> [_ _ _ _ _ w405 _ _ _ _ _ w424]
                tunnel: w383 -> [_ _ _ _ _ _ _ _ _ _ w417 _]
                tunnel: w373 -> [_ _ _ w401 _ _ _ _ _ _ _ _]
                frame #0 {
                  w398 = u16 3  # AcquisitionMode
                  n94 = call "SetAcquisitionMode.vi"("mode"=w398) -> ()  [unwired: 1 in, 2 out]
                }
                frame #1 {
                  w399 = u16 0  # ReadMode
                  n95 = call "SetReadMode.vi"("mode"=w399) -> ()  [unwired: 1 in, 2 out]
                }
                frame #2 {
                  n96 = call "SetTriggerMode.vi"("mode"=TriggerMode_mode_typedef."Internal") -> ()  [unwired: 1 in, 2 out]
                }
                frame #3 {
                  n97 = call "SetExposureTime.vi"("time"=w401) -> ()  [unwired: 1 in, 2 out]
                }
                frame #4 {
                  n98 = call "GetNumberVSSpeeds.vi"() -> ("number"=w404:i32)  [unwired: 3 in, 2 out]
                  n99 = Subtract(x=w404, y=1) -> (x-y=w402:i32)
                  n100 = call "SetVSSpeed.vi"("index"=w402) -> ()  [unwired: 1 in, 2 out]
                }
                frame #5 {
                  n101 = call "SetNumberKinetics.vi"("number"=w405) -> ()  [unwired: 1 in, 2 out]
                }
                frame #6 {
                  w409 = 0  # Auto Shutter
                  n102 = call "SetShutter.vi"("type"=Shutter_type_typedef."TTL High", "mode"=w409, "closingtime"=0, "openingtime"=0) -> ()  [unwired: 10 in, 2 out]
                }
                frame #7 {
                  n103 = call "GetAcquisitionTimings.vi"() -> ("exposure"=w410:sgl)  [unwired: 11 in, 4 out]
                  n104 = property on="Calculated exposure time" class="DigNum (strict)"("Value"=w410) -> ()  [unwired: 2 in, 2 out]
                }
                frame #8 {
                  n105 = call "StartAcquisition.vi"() -> ("DLL error code"=w411:u32)  [unwired: 2 in, 1 out]
                  n106 = property on="Start Aquisition return code" class="DigNum (strict)"("Value"=w411) -> ()  [unwired: 2 in, 2 out]
                }
                frame #9 {
                  n107 = while {
                    stop <- w414 continue-if-true
                    w415 = u16 72  # DRV ACQUIRING
                    n108 = call "GetStatus.vi"() -> ("DLL error code"=→"Get status return code":u32, "status"=w413:T19)  [unwired: 3 in, 1 out]
                    n109 = Equal?(x=w413, y=w415) -> (x = y?=w414:bool)
                  }
                }
                frame #10 {
                  n110 = flat-sequence {
                    tunnel: [w419] -> w418
                    tunnel: w417 -> [w419]
                    tunnel: [w423] -> w416
                    tunnel: w418 -> [w421]
                    frame #0 {
                    }
                    frame #1 {
                      n111 = call "GetAcquiredData.vi"("size"=w421) -> ("DLL error code"=w420:u32, "array"=w423:i32[])  [unwired: 2 in, 1 out]
                      n112 = Equal?(x=20002 ("DRV_SUCCESS"), y=w420) -> ()  [unwired: 1 out]
                      n113 = property on="get aquired data return code" class="DigNum (strict)"("Value"=w420) -> ()  [unwired: 2 in, 2 out]
                    }
                  }
                }
                frame #11 {
                  n114 = for {
                    N: w424 -> [_]
                    shift-right: [w428] -> w426
                    shift-left: i32[][] [] -> [w430]
                    tunnel: w425 -> [w429]
                    i -> [w433]
                    w431 = 1024 ("x")
                    n115 = Multiply(x=w431, y=w433) -> (x*y=w435:i32)
                    n116 = Equal To 0?(x=w433) -> (x = 0?=w434:bool)
                    n117 = Array Subset(array=w429, index=w435, length=w431) -> (w432:i32[])
                    n118 = case shown="False" w434 {
                      tunnel: w432 -> [w437 w440]
                      tunnel: w430 -> [w438 _]
                      tunnel: [w436 w439] -> w428
                      frame False {
                        n119 = Build Array (concatenate)(w438, w437) -> (w436:i32[][])
                      }
                      frame True {
                        n120 = Build Array(w440) -> (w439:i32[][])
                      }
                    }
                  }
                }
              }
              n121 = property on="Use autolab?" class="Bool (strict)"() -> ("Value"=w361:bool)  [unwired: 2 in, 2 out]
              n122 = case shown="True" w361 {
                tunnel: [SECenumctl."Apply potential" SECenumctl."Apply potential Autolab"] -> w360
                frame False {
                }
                frame True {
                }
              }
              n123 = Unbundle By Name(w365) -> ("Number of scans in kinetic cycle"=w367:i32)
              n124 = flat-sequence {
                tunnel: [w446] -> w363
                tunnel: w381 -> [w444]
                tunnel: w367 -> [w443]
                tunnel: [w441] -> w364
                frame #0 {
                  n125 = for {
                    N: 1023 -> [_]
                    tunnel: w444 -> [w451]
                    tunnel: [w452] -> w446 mode=indexing
                    tunnel: w443 -> [w449]
                    tunnel: [w447] -> w441 mode=indexing
                    i -> [w448]
                    n126 = Index Array(array=w451, index (col)=w448) -> (element=w450:i32[])  [unwired: 1 in]
                    n127 = Add Array Elements(numeric array=w450) -> (sum=w453:i32)
                    n128 = Increment(x=w448) -> (x+1=w447:i32)
                    n129 = Divide(x=w453, y=w449) -> (x/y=w452:dbl)
                  }
                  n130 = Bundle(w441, w446) -> (→"?":cluster{i32[], dbl[]})  [unwired: 1 in]
                }
              }
              n131 = case shown="True" w370 {
                tunnel: w369 -> [w388 _]
                tunnel: w363 -> [w387 w390]
                tunnel: [w386 w391] -> w368
                tunnel: w364 -> [_ w389]
                frame False {
                  n132 = Build Array (concatenate)(w388, w387) -> (w386:dbl[][])
                }
                frame True {
                  n133 = Build Array(w389, w390) -> (w391:dbl[][])
                }
              }
              n134 = case shown="False" w376 {
                selector: w376 -> [w392 w395]
                tunnel: [0.0 1.0] -> w378
                tunnel: [1.0 ("Stop \npotential") 0.0 ("Stop \npotential")] -> w377
                tunnel: [w392 w395] -> w375
                frame False {
                }
                frame True {
                }
              }
            }
            frame "Read spectrum from Ocean" {
              # "Building an matric of WL + intensities of multiple expts"
              n135 = Unbundle By Name(w463) -> ("Integration time"=w462:i32, "Continous strobe delay"=w461:i32)
              n136 = Equal?(x=w471, y=2) -> (x = y?=w469:bool)
              n137 = for {
                N: "Number of averages" -> [_]
                tunnel: [w485] -> w474
                tunnel: [w484] -> w468
                tunnel: w462 -> [w483]
                tunnel: w461 -> [w482]
                shift-right: [w479] -> w457
                shift-left: dbl[] [0.0, 0.0, 0.0, 0.0, 0.0, 0.0, 0.0, 0.0, 0.0, 0.0, 0.0, 0.0, 0.0, 0.0, 0.0, 0.0, 0.0, 0.0, 0.0, 0.0, 0.0, 0.0, 0.0, 0.0, 0.0, 0.0, 0.0, 0.0, 0.0, 0.0, 0.0, 0.0, 0.0, 0.0, 0.0, 0.0, 0.0, 0.0, 0.0, 0.0, 0.0, 0.0, 0.0, 0.0, 0.0, 0.0, 0.0, 0.0, 0.0, 0.0, 0.0, 0.0, 0.0, 0.0, 0.0, 0.0, 0.0, 0.0, 0.0, 0.0, 0.0, 0.0, 0.0, 0.0, 0.0, 0.0, 0.0, 0.0, 0.0, 0.0, 0.0, 0.0, 0.0, 0.0, 0.0, 0.0, 0.0, 0.0, 0.0, 0.0, 0.0, 0.0, 0.0, 0.0, 0.0, 0.0, 0.0, 0.0, 0.0, 0.0, 0.0, 0.0, 0.0, 0.0, 0.0, 0.0, 0.0, 0.0, 0.0, 0.0, 0.0, 0.0, 0.0, 0.0, 0.0, 0.0, 0.0, 0.0, 0.0, 0.0, 0.0, 0.0, 0.0, 0.0, 0.0, 0.0, 0.0, 0.0, 0.0, 0.0, 0.0, 0.0, 0.0, 0.0, 0.0, 0.0, 0.0, 0.0, 0.0, 0.0, 0.0, 0.0, 0.0, 0.0, 0.0, 0.0, 0.0, 0.0, 0.0, 0.0, 0.0, 0.0, 0.0, 0.0, 0.0, 0.0, 0.0, 0.0, 0.0, 0.0, 0.0, 0.0, 0.0, 0.0, 0.0, 0.0, 0.0, 0.0, 0.0, 0.0, 0.0, 0.0, 0.0, 0.0, 0.0, 0.0, 0.0, 0.0, 0.0, 0.0, 0.0, 0.0, 0.0, 0.0, 0.0, 0.0, 0.0, 0.0, 0.0, 0.0, 0.0, 0.0, 0.0, 0.0, 0.0, 0.0, 0.0, 0.0, 0.0, 0.0, 0.0, 0.0, 0.0, 0.0, 0.0, 0.0, 0.0, 0.0, 0.0, 0.0, 0.0, 0.0, 0.0, 0.0, 0.0, 0.0, 0.0, 0.0, 0.0, 0.0, 0.0, 0.0, 0.0, 0.0, 0.0, 0.0, 0.0, 0.0, 0.0, 0.0, 0.0, 0.0, 0.0, 0.0, 0.0, 0.0, 0.0, 0.0, 0.0, 0.0, 0.0, 0.0, 0.0, 0.0, 0.0, 0.0, 0.0, 0.0, 0.0, 0.0, 0.0, 0.0, 0.0, 0.0, 0.0, 0.0, 0.0, 0.0, 0.0, 0.0, 0.0, 0.0, 0.0, 0.0, 0.0, 0.0, 0.0, 0.0, 0.0, 0.0, 0.0, 0.0, 0.0, 0.0, 0.0, 0.0, 0.0, 0.0, 0.0, 0.0, 0.0, 0.0, 0.0, 0.0, 0.0, 0.0, 0.0, 0.0, 0.0, 0.0, 0.0, 0.0, 0.0, 0.0, 0.0, 0.0, 0.0, 0.0, 0.0, 0.0, 0.0, 0.0, 0.0, 0.0, 0.0, 0.0, 0.0, 0.0, 0.0, 0.0, 0.0, 0.0, 0.0, 0.0, 0.0, 0.0, 0.0, 0.0, 0.0, 0.0, 0.0, 0.0, 0.0, 0.0, 0.0, 0.0, 0.0, 0.0, 0.0, 0.0, 0.0, 0.0, 0.0, 0.0, 0.0, 0.0, 0.0, 0.0, 0.0, 0.0, 0.0, 0.0, 0.0, 0.0, 0.0, 0.0, 0.0, 0.0, 0.0, 0.0, 0.0, 0.0, 0.0, 0.0, 0.0, 0.0, 0.0, 0.0, 0.0, 0.0, 0.0, 0.0, 0.0, 0.0, 0.0, 0.0, 0.0, 0.0, 0.0, 0.0, 0.0, 0.0, 0.0, 0.0, 0.0, 0.0, 0.0, 0.0, 0.0, 0.0, 0.0, 0.0, 0.0, 0.0, 0.0, 0.0, 0.0, 0.0, 0.0, 0.0, 0.0, 0.0, 0.0, 0.0, 0.0, 0.0, 0.0, 0.0, 0.0, 0.0, 0.0, 0.0, 0.0, 0.0, 0.0, 0.0, 0.0, 0.0, 0.0, 0.0, 0.0, 0.0, 0.0, 0.0, 0.0, 0.0, 0.0, 0.0, 0.0, 0.0, 0.0, 0.0, 0.0, 0.0, 0.0, 0.0, 0.0, 0.0, 0.0, 0.0, 0.0, 0.0, 0.0, 0.0, 0.0, 0.0, 0.0, 0.0, 0.0, 0.0, 0.0, 0.0, 0.0, 0.0, 0.0, 0.0, 0.0, 0.0, 0.0, 0.0, 0.0, 0.0, 0.0, 0.0, 0.0, 0.0, 0.0, 0.0, 0.0, 0.0, 0.0, 0.0, 0.0, 0.0, 0.0, 0.0, 0.0, 0.0, 0.0, 0.0, 0.0, 0.0, 0.0, 0.0, 0.0, 0.0, 0.0, 0.0, 0.0, 0.0, 0.0, 0.0, 0.0, 0.0, 0.0, 0.0, 0.0, 0.0, 0.0, 0.0, 0.0, 0.0, 0.0, 0.0, 0.0, 0.0, 0.0, 0.0, 0.0, 0.0, 0.0, 0.0, 0.0, 0.0, 0.0, 0.0, 0.0, 0.0, 0.0, 0.0, 0.0, 0.0, 0.0, 0.0, 0.0, 0.0, 0.0, 0.0, 0.0, 0.0, 0.0, 0.0, 0.0, 0.0, 0.0, 0.0, 0.0, 0.0, 0.0, 0.0, 0.0, 0.0, 0.0, 0.0, 0.0, 0.0, 0.0, 0.0, 0.0, 0.0, 0.0, 0.0, 0.0, 0.0, 0.0, 0.0, 0.0, 0.0, 0.0, 0.0, 0.0, 0.0, 0.0, 0.0, 0.0, 0.0, 0.0, 0.0, 0.0, 0.0, 0.0, 0.0, 0.0, 0.0, 0.0, 0.0, 0.0, 0.0, 0.0, 0.0, 0.0, 0.0, 0.0, 0.0, 0.0, 0.0, 0.0, 0.0, 0.0, 0.0, 0.0, 0.0, 0.0, 0.0, 0.0, 0.0, 0.0, 0.0, 0.0, 0.0, 0.0, 0.0, 0.0, 0.0, 0.0, 0.0, 0.0, 0.0, 0.0, 0.0, 0.0, 0.0, 0.0, 0.0, 0.0, 0.0, 0.0, 0.0, 0.0, 0.0, 0.0, 0.0, 0.0, 0.0, 0.0, 0.0, 0.0, 0.0, 0.0, 0.0, 0.0, 0.0, 0.0, 0.0, 0.0, 0.0, 0.0, 0.0, 0.0, 0.0, 0.0, 0.0, 0.0, 0.0, 0.0, 0.0, 0.0, 0.0, 0.0, 0.0, 0.0, 0.0, 0.0, 0.0, 0.0, 0.0, 0.0, 0.0, 0.0, 0.0, 0.0, 0.0, 0.0, 0.0, 0.0, 0.0, 0.0, 0.0, 0.0, 0.0, 0.0, 0.0, 0.0, 0.0, 0.0, 0.0, 0.0, 0.0, 0.0, 0.0, 0.0, 0.0, 0.0, 0.0, 0.0, 0.0, 0.0, 0.0, 0.0, 0.0, 0.0, 0.0, 0.0, 0.0, 0.0, 0.0, 0.0, 0.0, 0.0, 0.0, 0.0, 0.0, 0.0, 0.0, 0.0, 0.0, 0.0, 0.0, 0.0, 0.0, 0.0, 0.0, 0.0, 0.0, 0.0, 0.0, 0.0, 0.0, 0.0, 0.0, 0.0, 0.0, 0.0, 0.0, 0.0, 0.0, 0.0, 0.0, 0.0, 0.0, 0.0, 0.0, 0.0, 0.0, 0.0, 0.0, 0.0, 0.0, 0.0, 0.0, 0.0, 0.0, 0.0, 0.0, 0.0, 0.0, 0.0, 0.0, 0.0, 0.0, 0.0, 0.0, 0.0, 0.0, 0.0, 0.0, 0.0, 0.0, 0.0, 0.0, 0.0, 0.0, 0.0, 0.0, 0.0, 0.0, 0.0, 0.0, 0.0, 0.0, 0.0, 0.0, 0.0, 0.0, 0.0, 0.0, 0.0, 0.0, 0.0, 0.0, 0.0, 0.0, 0.0, 0.0, 0.0, 0.0, 0.0, 0.0, 0.0, 0.0, 0.0, 0.0, 0.0, 0.0, 0.0, 0.0, 0.0, 0.0, 0.0, 0.0, 0.0, 0.0, 0.0, 0.0, 0.0, 0.0, 0.0, 0.0, 0.0, 0.0, 0.0, 0.0, 0.0, 0.0, 0.0, 0.0, 0.0, 0.0, 0.0, 0.0, 0.0, 0.0, 0.0, 0.0, 0.0, 0.0, 0.0, 0.0, 0.0, 0.0, 0.0, 0.0, 0.0, 0.0, 0.0, 0.0, 0.0, 0.0, 0.0, 0.0, 0.0, 0.0, 0.0, 0.0, 0.0, 0.0, 0.0, 0.0, 0.0, 0.0, 0.0, 0.0, 0.0, 0.0, 0.0, 0.0, 0.0, 0.0, 0.0, 0.0, 0.0, 0.0, 0.0, 0.0, 0.0, 0.0, 0.0, 0.0, 0.0, 0.0, 0.0, 0.0, 0.0, 0.0, 0.0, 0.0, 0.0, 0.0, 0.0, 0.0, 0.0, 0.0, 0.0, 0.0, 0.0, 0.0, 0.0, 0.0, 0.0, 0.0, 0.0, 0.0, 0.0, 0.0, 0.0, 0.0, 0.0, 0.0, 0.0, 0.0, 0.0, 0.0, 0.0, 0.0, 0.0, 0.0, 0.0, 0.0, 0.0, 0.0, 0.0, 0.0, 0.0, 0.0, 0.0, 0.0, 0.0, 0.0, 0.0, 0.0, 0.0, 0.0, 0.0, 0.0, 0.0, 0.0, 0.0, 0.0, 0.0, 0.0, 0.0, 0.0, 0.0, 0.0, 0.0, 0.0, 0.0, 0.0, 0.0, 0.0, 0.0, 0.0, 0.0, 0.0, 0.0, 0.0, 0.0, 0.0, 0.0, 0.0, 0.0, 0.0, 0.0, 0.0, 0.0, 0.0, 0.0, 0.0, 0.0, 0.0, 0.0, 0.0, 0.0, 0.0, 0.0, 0.0, 0.0, 0.0, 0.0, 0.0, 0.0, 0.0, 0.0, 0.0, 0.0, 0.0, 0.0, 0.0, 0.0, 0.0, 0.0, 0.0, 0.0, 0.0, 0.0, 0.0, 0.0, 0.0, 0.0, 0.0, 0.0, 0.0, 0.0, 0.0, 0.0, 0.0, 0.0, 0.0, 0.0, 0.0, 0.0, 0.0, 0.0, 0.0, 0.0, 0.0, 0.0, 0.0, 0.0, 0.0, 0.0, 0.0, 0.0, 0.0, 0.0, 0.0, 0.0, 0.0, 0.0, 0.0, 0.0, 0.0, 0.0, 0.0, 0.0, 0.0, 0.0, 0.0, 0.0, 0.0, 0.0, 0.0, 0.0, 0.0, 0.0, 0.0, 0.0, 0.0, 0.0, 0.0, 0.0, 0.0, 0.0, 0.0, 0.0] -> [w480]
                i -> [w478]
                n138 = call "ReadSpectrum(SubVI).vi"("Continuous \nStrobe Delay"=w482, "Enter the \nInetegration Time"=w483) -> ("Spectrum Values"=w481:dbl[], "WL Values"=w484:dbl[], "Number of Spectrometers"=w485:i32)  [unwired: 7 in]
                n139 = Add(x=w481, y=w480) -> (x+y=w479:dbl[])
                "Number of time the OCEAN averaging loop has run -1" <- w478
              }
              "Number of Spectrometers" <- w474
              n140 = Divide(x=w457, y="Number of averages") -> (x/y=w456:dbl[])
              n141 = case shown="False" w469 {
                tunnel: w468 -> [_ w497]
                tunnel: w456 -> [w493 w496]
                tunnel: [w492 w495] -> w466
                tunnel: w465 -> [w494 _]
                frame False {
                  # "Matrix + int on i >3"
                  n142 = Build Array (concatenate)(w494, w493) -> (w492:dbl[][])
                }
                frame True {
                  # "WL + Int on =3"
                  n143 = Build Array(w497, w496) -> (w495:dbl[][])
                }
              }
              n144 = Bundle("WL Values"=w468, w456) -> (→"?":cluster{"WL Values":dbl[], dbl[]})  [unwired: 1 in]
              n145 = property on="Use autolab?" class="Bool (strict)"() -> ("Value"=w458:bool)  [unwired: 2 in, 2 out]
              n146 = case shown="True" w458 {
                tunnel: [SECenumctl."Apply potential" SECenumctl."Apply potential Autolab"] -> w459
                frame False {
                }
                frame True {
                }
              }
              n147 = case shown="False" w464 {
                tunnel: [0.0 1.0] -> w477
                tunnel: [1.0 ("Stop \npotential") 0.0 ("Stop \npotential")] -> w476
                frame False {
                }
                frame True {
                }
              }
            }
          }
          n148 = case shown="False" w209 {
            tunnel: w221 -> [w231 w233]
            tunnel: w219 -> [w230 w232]
            tunnel: [w229 w234] -> w208
            frame False {
              n149 = Greater Or Equal?(x=w231, y=w230) -> (x >= y?=w229:bool)
            }
            frame True {
              n150 = Less Or Equal?(x=w233, y=w232) -> (x <= y?=w234:bool)
            }
          }
        }
        n151 = Unbundle By Name(w158) -> ("Default\n potential"=w179:dbl)
        n152 = property on="Use autolab?" class="Bool (strict)"() -> ("Value"=w153:bool)  [unwired: 2 in, 2 out]
        n153 = Insert Into Array(array=w160, index=0, new element=0.0 ("new element/subarray")) -> (w169:dbl[])
        n154 = Transpose Matrix(1:w173) -> (0:w172:dbl[][])
        n155 = Bundle(w160, w164) -> (→"?":cluster{dbl[], dbl[]})  [unwired: 1 in]
        n156 = Reverse 1D Array(array=w169) -> (reversed array=w168:dbl[])
        n157 = property on="V (during measurment)" class="DigNum (strict)"("Value"=w179) -> ()  [unwired: 2 in, 2 out]
        n158 = case shown="True" w153 {
          tunnel: w179 -> [w187 w189]
          frame False {
            n159 = call "IV setpotential.vi"("value"=w187) -> ()  [unwired: 8 in, 3 out]
          }
          frame True {
            n160 = property on="Ei" class="Ref (strict)"() -> ("Value"=w188:refnum<k24>)  [unwired: 2 in, 2 out]
            n161 = property class="EI"(reference=w188, "Setpoint"=w189) -> ()  [unwired: 1 in, 2 out]
          }
        }
        n162 = Replace Array Subset(array=w172, new element=w168, index (row)=0 ("index")) -> (w157:dbl[][])  [unwired: 1 in]
        n163 = Bundle By Name(cluster=w158, "Spectrum"=w172, "Current array"=w164, "Potential array"=w160) -> (w159:T11)
        n164 = Build Array(w160, w164) -> (w171:dbl[][])
        n165 = disable-structure shown="Enabled" {
          disable-tunnel: w157 -> [w205 _]
          disable-tunnel: w158 -> [w204 _]
          frame Enabled {
            n166 = call "WriteSEC.vi"("Init cluster"=w204, "Array"=w205) -> ()  [unwired: 10 in]
          }
          frame Disabled {
          }
        }
        n167 = Transpose Matrix(1:w171) -> (0:w170:dbl[][])
        n168 = disable-structure shown="Enabled" {
          disable-tunnel: w170 -> [w203 _]
          disable-tunnel: w159 -> [w202 _]
          frame Enabled {
            n169 = call "Write_JV.vi"("Init cluster"=w202, "Array"=w203) -> ()  [unwired: 10 in]
          }
          frame Disabled {
          }
        }
      }
      frame "Exit" {
        w501 = TRUE  # Stop Loop?
        w504 = State."Exit"  # (Value Not Used)
        # "Switch cell on/off"
        # "Diconnect device and close Ivium remdriver"
        # "Disconnect Ivium device (when connected)\nbefore terminating this VI"
        # "Exit - Exit the application."
        n170 = property on="Shut down sequence run?" class="Bool (strict)"("Value"=FALSE ("Shut down sequence run?")) -> ()  [unwired: 2 in, 2 out]
        n171 = property on="PotentialOverload" class="Bool (strict)"("Value"=FALSE ("PotentialOverload")) -> ()  [unwired: 2 in, 2 out]
        n172 = property on="T reached?" class="Bool (strict)"("Value"=FALSE ("T reached?")) -> ()  [unwired: 2 in, 2 out]
        n173 = property on="Use autolab?" class="Bool (strict)"() -> ("Value"=w502:bool)  [unwired: 2 in, 2 out]
        n174 = case shown="True" w502 {
          tunnel: [w516 w534] -> w508
          tunnel: w507 -> [w513 w529]
          tunnel: [w511 0 ("devconnect")] -> w506
          frame False {
            w509 = FALSE ("Shut down sequence run?")
            # "This re-initialises a display for the iDus camera"
            # "On"
            # "Close Ivium Driver"
            n175 = To Long Integer(number=0) -> (32bit integer=w515:i32)
            n176 = call "IV setcellon.vi"("error in (no error)"=w513, "cellon"=w515) -> ("error out"=w512:errorcluster)  [unwired: 7 in, 2 out]
            n177 = call "IV getdevicestatus.vi"("error in (no error)"=w512) -> ("error out"=w517:errorcluster, "return type"=w518:i32)  [unwired: 9 in]
            n178 = Greater Than 0?(x=w518) -> (x > 0?=w510:bool)
            n179 = case shown="False" w510 {
              tunnel: [w521 w523] -> w519
              tunnel: w517 -> [w521 _]
              tunnel: [0 ("devconnect") w522] -> w511
              frame False {
              }
              frame True {
                w522 = 0 ("devconnect")
                n180 = call "IV connect.vi"("devconnect"=w522) -> ("error out"=w523:errorcluster)  [unwired: 8 in, 2 out]
              }
            }
            n181 = property on="Shut down sequence run?" class="Bool (strict)"("Value"=w509) -> ()  [unwired: 2 in, 2 out]
            n182 = property on="Return detector \nto room T?" class="Bool (strict)"("Value"=w509) -> ()  [unwired: 2 in, 2 out]
            n183 = call "IV close.vi"("error in (no error)"=w519) -> ("error out"=w516:errorcluster)  [unwired: 9 in, 1 out]
          }
          frame True {
            w528 = 0 items=["Off", "On"] ("CellOnOff")
            n184 = property on="Ei" class="Ref (strict)"() -> ("Value"=w527:refnum<k24>)  [unwired: 2 in, 2 out]
            n185 = property class="EI"(reference=w527, error in=w529, "CellOnOff"=w528) -> (error out=w526:errorcluster)  [unwired: 1 out]
            n186 = property on="ManualCellSwitch" class="Bool (strict)"("Value"=FALSE ("ManualCellSwitch")) -> ()  [unwired: 2 in, 2 out]
            n187 = property on="Cell on?" class="Bool (strict)"("Value"=FALSE ("Cell")) -> ()  [unwired: 2 in, 2 out]
            n188 = property on="instrument" class="Ref (strict)"(error in=w526) -> (error out=w532:errorcluster, "Value"=w533:refnum<k24>)  [unwired: 1 in, 1 out]
            n189 = property on="Autolab Connected?" class="Bool (strict)"("Value"=FALSE ("IsConnected")) -> ()  [unwired: 2 in, 2 out]
            n190 = invoke class="Instrument" method="Disconnect"(reference=w533, error in=w532) -> (error out=w534:errorcluster)  [unwired: 1 in, 2 out]
          }
        }
        n191 = property on="V2 applied?" class="Bool (strict)"("Value"=FALSE ("V2 applied")) -> ()  [unwired: 2 in, 2 out]
      }
      frame "Run OSPEC" {
        n192 = property on="Use autolab?" class="Bool (strict)"() -> ("Value"=w536:bool)  [unwired: 2 in, 2 out]
        n193 = case shown="True" w536 {
          tunnel: w543 -> [w549 w557]
          tunnel: [w548 w557] -> w542
          frame False {
            # "Get cell status"
            # "Get Device Status"
            # "Direct Mode"
            n194 = call "IV getdevicestatus.vi"() -> ("return type"=w552:i32)  [unwired: 10 in, 1 out]
            n195 = Increment(x=w552) -> (x+1=w551:i32)
            n196 = case shown="0, Default" w551 {
              tunnel: ["no IviumSoft" "device not connected" "device available_idle" "device available_busy"] -> w550
              frame 0, Default {
              }
              frame 1 {
              }
              frame 2 {
              }
              frame 3 {
              }
            }
            n197 = Bundle By Name(cluster=w549, "Status"=w550) -> (w548:T11)
          }
          frame True {
          }
        }
        n198 = while {
          shift-right: [w558] -> w540
          shift-left: w541 -> [w563]
          shift-right: [w559] -> w539
          shift-left: w542 -> [w565]
          shift-right: [w562] -> _
          shift-left: OSSPEC."Apply V1" -> [w564]
          i -> [w561]
          stop <- w560 stop-if-true
          n199 = case shown="\"Read current and spectrum\"" w564 {
            tunnel: w565 -> [w569 w956 w1486 w1510 w1572 w1635]
            tunnel: w563 -> [w568 w972 w1490 w1509 w1582 w1663]
            tunnel: [OSSPEC."End measurment" w988 OSSPEC."Read Potential and spectrum" OSSPEC."Read current and spectrum" OSSPEC."Read current and spectrum" OSSPEC."End measurment"] -> w562
            tunnel: [w574 w971 w1489 w1505 w1573 w1661] -> w558
            tunnel: [w575 w979 w1486 w1506 w1572 w1635] -> w559
            tunnel: w561 -> [_ _ _ _ _ _]
            tunnel: [FALSE FALSE FALSE FALSE FALSE w1662] -> w560
            frame "Read Potential and spectrum", Default {
              n200 = property on="Use autolab?" class="Bool (strict)"() -> ("Value"=w566:bool)  [unwired: 2 in, 2 out]
              n201 = disable-structure shown="Enabled" {
                disable-tunnel: w568 -> [w590 _]
                disable-tunnel: [w589 _] -> w567
                disable-tunnel: w566 -> [w588 _]
                frame Enabled {
                  n202 = case shown="True" w588 {
                    tunnel: w590 -> [w592 w604]
                    tunnel: [w591 w602] -> w589
                    frame False {
                      n203 = flat-sequence {
                        tunnel: w592 -> [w595]
                        tunnel: [w595] -> w593
                        tunnel: [w596] -> w591
                        tunnel: w593 -> [w597]
                        frame #0 {
                          n204 = Wait (ms)(milliseconds to wait=u32 50) -> ()  [unwired: 1 out]
                        }
                        frame #1 {
                          n205 = To Long Integer(number=T17."IStat4EL" ("Configuration")) -> (32bit integer=w599:i32)
                          n206 = call "IV setconnectionmode.vi"("error in (no error)"=w597, "value"=w599) -> ("error out"=w596:errorcluster)  [unwired: 7 in, 2 out]
                        }
                      }
                    }
                    frame True {
                      w600 = 0 items=["Off", "On"] ("CellOnOff")
                      w605 = -6 items=["CR07_1A"=0, "CR06_10A"=1, "CR01_100A"=2, "CR00_1000A"=3, "CR05_20A"=20, "CR04_40A"=40, "CR03_50A"=60, "CR02_80A"=80, "CR19_1pA"=-12, "CR18_10pA"=-11, "CR17_100pA"=-10, "CR16_1nA"=-9, "CR15_10nA"=-8, "CR14_100nA"=-7, "CR13_1uA"=-6, "CR12_10uA"=-5, "CR11_100uA"=-4, "CR10_1mA"=-3, "CR09_10mA"=-2, "CR08_100mA"=-1] ("CurrentRange")
                      w606 = 1 items=["Potentiostatic", "Galvanostatic"] ("Mode")
                      n207 = property on="Ei" class="Ref (strict)"() -> ("Value"=w601:refnum<k24>)  [unwired: 2 in, 2 out]
                      n208 = property class="EI"(reference=w601, error in=w604, "CurrentRange"=w605) -> (error out=w603:errorcluster)  [unwired: 1 out]
                      n209 = property class="EI"(reference=w601, error in=w603, "Mode"=w606, "CellOnOff"=w600) -> (error out=w602:errorcluster)  [unwired: 1 out]
                    }
                  }
                }
                frame Disabled {
                }
              }
              n210 = Unbundle By Name(w569) -> ("Spectrum"=w577:dbl[][])
              n211 = Unbundle By Name(w569) -> ("Time for spectrum measurment"=w576:i32[], "Start time"=w579:i32)
              n212 = Unbundle By Name(w569) -> ("Potential array"=w572:dbl[])
              n213 = property on="Use iDus?" class="Bool (strict)"() -> ("Value"=w570:bool)  [unwired: 2 in, 2 out]
              n214 = Unbundle By Name(w569) -> ("Time for E measurment"=w571:i32[], "Start time"=w578:i32)
              n215 = while {
                shift-right: [w838] -> _
                shift-left: w569 -> [w839]
                shift-right: [w830] -> _
                shift-left: OSPEC-enum."Wait" -> [w840]
                shift-right: [w837] -> w582
                shift-left: w571 -> [w836]
                shift-right: [w831] -> w581
                shift-left: w572 -> [w834]
                shift-right: [w833] -> _
                shift-left: w578 -> [w832]
                shift-right: [w828] -> w574
                shift-left: w567 -> [w829]
                i -> [w835]
                stop <- w825 stop-if-true
                n216 = case shown="\"Read\", Default" w840 {
                  tunnel: w839 -> [w848 w859 w950]
                  tunnel: [w848 w859 w950] -> w838
                  tunnel: [w847 FALSE FALSE] -> w827
                  tunnel: [w852 w863 w948] -> w837
                  tunnel: w836 -> [w852 w864 w948]
                  tunnel: w835 -> [_ w868 _]
                  tunnel: [w850 w867 w945] -> w831
                  tunnel: w834 -> [w850 w866 w945]
                  tunnel: [w843 w860 w947] -> w833
                  tunnel: w832 -> [w843 _ w947]
                  tunnel: [OSPEC-enum."Wait" OSPEC-enum."Check exit" OSPEC-enum."Read"] -> w830
                  tunnel: w829 -> [w849 w856 w944]
                  tunnel: [w849 w855 w944] -> w828
                  frame "Check exit" {
                    n217 = Unbundle By Name(w848) -> ("V off time"=w845:dbl)
                    n218 = Multiply(x=w845, y=1000.0) -> (x*y=w846:dbl)
                    n219 = Greater Or Equal?(x=w843, y=w846) -> (x >= y?=w847:bool)
                  }
                  frame "Read", Default {
                    # "Building a 1d matrix of potentials and times"
                    n220 = property on="Use autolab?" class="Bool (strict)"() -> ("Value"=w853:bool)  [unwired: 2 in, 2 out]
                    n221 = case shown="True" w853 {
                      tunnel: [w871 w874] -> w857
                      tunnel: w856 -> [w870 w872]
                      tunnel: [w869 w873] -> w855
                      frame False {
                        n222 = call "IV getpotential.vi"("error in (no error)"=w870) -> ("error out"=w869:errorcluster, "value out"=w871:dbl)  [unwired: 8 in, 1 out]
                      }
                      frame True {
                        n223 = disable-structure shown="Enabled" {
                          disable-tunnel: [w879 _ w925] -> w874
                          disable-tunnel: [w878 _ w927] -> w873
                          disable-tunnel: w872 -> [w876 _ w935]
                          frame Disabled {
                            n224 = property on="Ei" class="Ref (strict)"() -> ("Value"=w877:refnum<k24>)  [unwired: 2 in, 2 out]
                            n225 = disable-structure shown="Enabled" {
                              disable-tunnel: w877 -> [w887 _]
                              disable-tunnel: w876 -> [w883 w888]
                              disable-tunnel: [w882 w888] -> w875
                              frame Disabled {
                                w884 = -4 items=["CR07_1A"=0, "CR06_10A"=1, "CR01_100A"=2, "CR00_1000A"=3, "CR05_20A"=20, "CR04_40A"=40, "CR03_50A"=60, "CR02_80A"=80, "CR19_1pA"=-12, "CR18_10pA"=-11, "CR17_100pA"=-10, "CR16_1nA"=-9, "CR15_10nA"=-8, "CR14_100nA"=-7, "CR13_1uA"=-6, "CR12_10uA"=-5, "CR11_100uA"=-4, "CR10_1mA"=-3, "CR09_10mA"=-2, "CR08_100mA"=-1] ("CurrentRange")
                                w886 = 1 items=["Potentiostatic", "Galvanostatic"] ("Mode")
                                n226 = property class="EI"(reference=w887, error in=w883, "Mode"=w886, "Setpoint"=0.0, "CurrentRange"=w884) -> (error out=w882:errorcluster)  [unwired: 1 out]
                              }
                              frame Enabled {
                              }
                            }
                            n227 = property class="EI"(reference=w877, error in=w875) -> (error out=w878:errorcluster, "Current"=w880:dbl, "Potential"=w879:dbl)  [unwired: 1 out]
                            n228 = disable-structure shown="Enabled" {
                              disable-tunnel: w880 -> [w881 _]
                              frame Disabled {
                                "OCP I (close to 0)" <- w881
                              }
                              frame Enabled {
                              }
                            }
                          }
                          frame Disabled {
                            n229 = property on="Property Node" class="Ref (strict)"() -> ("Value"=w890:refnum<k24>)  [unwired: 2 in, 2 out]
                            n230 = disable-structure shown="Disabled" {
                              disable-tunnel: _ -> [w916 _]
                              disable-tunnel: [w915 _] -> _
                              disable-tunnel: _ -> [w912 _]
                              disable-tunnel: w890 -> [w911 _]
                              frame Disabled {
                                w909 = 2 items=["UltraHigh_Speed", "High_Speed", "High_Stability"] ("Bandwidth")
                                w914 = 1 items=["Off", "On"] ("CellOnOff")
                                w910 = 0 items=["Potentiostatic", "Galvanostatic"] ("Mode")
                                n231 = property on="Property Node" class="Ring (strict)"() -> ("Value"=w913:i32)  [unwired: 2 in, 2 out]
                                n232 = property class="EI"(reference=w911, error in=w912, "Bandwidth"=w909, "CellOnOff"=w914, "CurrentRange"=w913, "Mode"=w910, "Setpoint"=w916) -> (error out=w915:errorcluster)  [unwired: 1 out]
                                n233 = property on="Property Node" class="Ref (strict)"(error in=w915) -> (error out=w908:errorcluster, "Value"=w905:refnum<k24>)  [unwired: 1 in, 1 out]
                                n234 = property class="EI"(reference=w911, error in=w915) -> (error out=w906:errorcluster, "EiStatusSupportedFor"=w907:string[])  [unwired: 1 out]
                                n235 = invoke class="Sampler" method="Sample"(reference=w905, error in=w908) -> ()  [unwired: 1 in, 3 out]
                                n236 = property on="Property Node" class="Arr (strict)"(error in=w906, "Value"=w907) -> ()  [unwired: 1 in, 2 out]
                              }
                              frame Enabled {
                              }
                            }
                            n237 = property class="EI"(reference=w890) -> (error in=w892:errorcluster, error out=w891:errorcluster, "Setpoint"=w889:dbl)  [unwired: 1 out]
                            n238 = property class="EI" props=["Bandwidth", "CurrentRange", "Mode", "Setpoint", "Current", "Potential"](reference=w890, error in=w891) -> (error out=w893:errorcluster, "Bandwidth"=w904:i32, "CurrentRange"=w903:i32, "Mode"=w902:i32, "Current"=w896:dbl, "Potential"=w895:dbl)  [unwired: 2 out]
                            n239 = property on="Property Node" class="Ring (strict)"("Value"=w904) -> ()  [unwired: 2 in, 2 out]
                            n240 = property on="Property Node" class="Ring (strict)"("Value"=w903) -> ()  [unwired: 2 in, 2 out]
                            n241 = property on="Property Node" class="Ring (strict)"("Value"=w902) -> ()  [unwired: 2 in, 2 out]
                            n242 = flat-sequence {
                              tunnel: [w920] -> w901
                              tunnel: w896 -> [w919]
                              tunnel: w895 -> [w918]
                              tunnel: [w917] -> w894
                              tunnel: w893 -> [w917]
                              frame #0 {
                                n243 = call "Range_selector.vi"("potential"=w918, "current"=w919) -> ("range integer"=w920:i32)  [unwired: 9 in]
                              }
                            }
                            n244 = property class="EI"(reference=w890, error in=w894) -> (error out=w900:errorcluster, "Current"=→"Current PD 2":dbl, "Potential"=→"POtential PD 2":dbl)  [unwired: 1 out]
                            n245 = property class="EI"(reference=w890, error in=w900, "CurrentRange"=w901) -> (error out=w899:errorcluster)  [unwired: 1 out]
                          }
                          frame Enabled {
                            w922 = -9 items=["CR07_1A"=0, "CR06_10A"=1, "CR01_100A"=2, "CR00_1000A"=3, "CR05_20A"=20, "CR04_40A"=40, "CR03_50A"=60, "CR02_80A"=80, "CR19_1pA"=-12, "CR18_10pA"=-11, "CR17_100pA"=-10, "CR16_1nA"=-9, "CR15_10nA"=-8, "CR14_100nA"=-7, "CR13_1uA"=-6, "CR12_10uA"=-5, "CR11_100uA"=-4, "CR10_1mA"=-3, "CR09_10mA"=-2, "CR08_100mA"=-1] ("CurrentRange")
                            w932 = -9 items=["CR07_1A"=0, "CR06_10A"=1, "CR01_100A"=2, "CR00_1000A"=3, "CR05_20A"=20, "CR04_40A"=40, "CR03_50A"=60, "CR02_80A"=80, "CR19_1pA"=-12, "CR18_10pA"=-11, "CR17_100pA"=-10, "CR16_1nA"=-9, "CR15_10nA"=-8, "CR14_100nA"=-7, "CR13_1uA"=-6, "CR12_10uA"=-5, "CR11_100uA"=-4, "CR10_1mA"=-3, "CR09_10mA"=-2, "CR08_100mA"=-1] ("CurrentRange")
                            w936 = 0 items=["Off", "On"] ("CellOnOff")
                            w937 = 2 items=["UltraHigh_Speed", "High_Speed", "High_Stability"] ("Bandwidth")
                            w938 = 1 items=["Potentiostatic", "Galvanostatic"] ("Mode")
                            w942 = 1 items=["Potentiostatic", "Galvanostatic"] ("Mode")
                            w924 = 0 items=["Off", "On"] ("CellOnOff")
                            w943 = 2 items=["UltraHigh_Speed", "High_Speed", "High_Stability"] ("Bandwidth")
                            n246 = property on="Ei" class="Ref (strict)"() -> ("Value"=w934:refnum<k24>)  [unwired: 2 in, 2 out]
                            n247 = property on="Sampler 2" class="Ref (strict)"() -> ("Value"=w933:refnum<k24>)  [unwired: 2 in, 2 out]
                            n248 = call "EI (A).vi"("Sampler"=w933, "Ei"=w934, "CellOnOff"=w924, "Setpoint"=0.0, "Bandwidth"=w943, "CurrentRange"=w932, "Mode"=w942, "error in (no error)"=w935, "Disable Sampler"=FALSE) -> ("Cell"=w931:bool, "PotentialOverload"=w930:bool, "Setpoint"=→"Setpoint":dbl, "error out"=w928:errorcluster)  [unwired: 5 in, 10 out]
                            n249 = property on="PotentialOverload" class="Bool (strict)"("Value"=w930) -> ()  [unwired: 2 in, 2 out]
                            n250 = property on="Cell on?" class="Bool (strict)"("Value"=w931) -> ()  [unwired: 2 in, 2 out]
                            n251 = call "Sampler.vi"("error in (no error)"=w935, "Sampler"=w933) -> ("error out"=w940:errorcluster)  [unwired: 7 in, 2 out]
                            n252 = Merge Errors(w940, w928) -> (w941:errorcluster)
                            n253 = call "EI (A).vi"("Sampler"=w933, "Ei"=w934, "CellOnOff"=w936, "Bandwidth"=w937, "CurrentRange"=w922, "Mode"=w938, "error in (no error)"=w941, "Disable Sampler"=FALSE) -> ("Potential"=w925:dbl, "Current"=w926:dbl, "error out"=w927:errorcluster)  [unwired: 6 in, 11 out]
                            "Potential  During PD" <- w925
                            n254 = property on="current" class="DigNum (strict)"("Value"=w926) -> ()  [unwired: 2 in, 2 out]
                            n255 = property on="Voltage" class="DigNum (strict)"("Value"=w925) -> ()  [unwired: 2 in, 2 out]
                          }
                        }
                      }
                    }
                    "OCP" <- w857
                    n256 = Unbundle By Name(w859) -> ("Start time"=w858:i32)
                    n257 = Tick Count (ms)() -> (millisecond timer value=w854:u32)
                    n258 = Subtract(x=w854, y=w858) -> (x-y=w860:u32)
                    n259 = Equal?(x=1, y=w868) -> ()  [unwired: 1 out]
                    n260 = Build Array (concatenate)(w864, w860) -> (w863:u32[])
                    n261 = Build Array (concatenate)(w866, w857) -> (w867:dbl[])
                  }
                  frame "Wait" {
                    n262 = Unbundle By Name(w950) -> ("Sample rate"=w951:dbl)
                    n263 = Multiply(x=w951, y=1000.0) -> (x*y=w953:dbl)
                    n264 = Wait (ms)(milliseconds to wait=w953) -> ()  [unwired: 1 out]
                  }
                }
                n265 = property on="Use iDus?" class="Bool (strict)"() -> ("Value"=w824:bool)  [unwired: 2 in, 2 out]
                n266 = case shown="False" w824 {
                  tunnel: [TRUE ("Value") w842] -> w826
                  frame False {
                  }
                  frame True {
                    n267 = property on="IDus not in read loop? (kinetic)" class="Bool (strict)"() -> ("Value"=w842:bool)  [unwired: 2 in, 2 out]
                  }
                }
                n268 = And(x=w826, y=w827) -> (x .and. y?=w825:bool)
              }
              n269 = case shown="False" w570 {
                tunnel: [w620 w699] -> w584
                tunnel: [w619 w700] -> w583
                tunnel: w579 -> [w618 w706]
                tunnel: w577 -> [w617 w704]
                tunnel: w576 -> [w616 w702]
                tunnel: [w615 w701] -> w573
                tunnel: w569 -> [w614 w705]
                frame False {
                  n270 = disable-structure shown="Enabled" {
                    disable-tunnel: w614 -> [w632 _]
                    disable-tunnel: [w629 w633] -> w613
                    disable-tunnel: [w628 w635] -> w612
                    disable-tunnel: [w627 w634] -> w611
                    frame Disabled {
                      n271 = Unbundle By Name(w632) -> ("Continous strobe delay"=w630:i32, "Integration time"=w631:i32)
                      n272 = call "OSPEC-Open-Ocean.vi"("Integration Time"=w630, "delay"=w631) -> ("WL Values"=w629:dbl[], "Wrapper Out"=w627:u32, "ContinuousStrobe Out"=w628:u32)  [unwired: 7 in]
                    }
                    frame Enabled {
                      n273 = property on="WL Values" class="Arr (strict)"() -> ("Value"=w633:dbl[])  [unwired: 2 in, 2 out]
                      n274 = property on="ContinuousStrobe Out" class="DigNum (strict)"() -> ("Value"=w635:u32)  [unwired: 2 in, 2 out]
                      n275 = property on="Wrapper Out" class="DigNum (strict)"() -> ("Value"=w634:u32)  [unwired: 2 in, 2 out]
                    }
                  }
                  n276 = while {
                    shift-right: [w650] -> _
                    shift-left: w614 -> [w651]
                    shift-right: [w643] -> _
                    shift-left: OSPEC-enum."Read" -> [w652]
                    shift-right: [w648] -> w619
                    shift-left: w616 -> [w647]
                    shift-right: [w642] -> w615
                    shift-left: w617 -> [w646]
                    shift-right: [w645] -> w620
                    shift-left: w618 -> [w639]
                    tunnel: w611 -> [w641]
                    tunnel: [w640] -> w608
                    tunnel: w613 -> [w638]
                    tunnel: [w637] -> w607
                    tunnel: w612 -> [w636]
                    i -> [w644]
                    stop <- w649 stop-if-true
                    n277 = case shown="\"Wait\"" w652 {
                      tunnel: w651 -> [w662 w674 w693]
                      tunnel: [w662 w674 w693] -> w650
                      tunnel: [w661 FALSE FALSE] -> w649
                      tunnel: [w664 w680 w691] -> w648
                      tunnel: w647 -> [w664 w679 w691]
                      tunnel: w644 -> [_ _ _]
                      tunnel: [w660 w675 w687] -> w642
                      tunnel: w646 -> [w660 w678 w687]
                      tunnel: [w653 w671 w684] -> w645
                      tunnel: w639 -> [w653 _ w684]
                      tunnel: [OSPEC-enum."Wait" OSPEC-enum."Check exit" OSPEC-enum."Read"] -> w643
                      tunnel: w641 -> [w658 w665 w688]
                      tunnel: [w659 w670 w689] -> _
                      tunnel: w638 -> [w659 w670 w689]
                      tunnel: [w658 w665 w688] -> w640
                      tunnel: [w655 w668 w682] -> w637
                      tunnel: w636 -> [w655 w668 w682]
                      frame "Check exit" {
                        n278 = Unbundle By Name(w662) -> ("V off time"=w657:dbl)
                        n279 = Multiply(x=w657, y=1000.0) -> (x*y=w654:dbl)
                        n280 = Greater Or Equal?(x=w653, y=w654) -> (x >= y?=w661:bool)
                      }
                      frame "Read", Default {
                        # "Continue 2d matrix of specta"
                        # "Continue to add times to this"
                        n281 = Tick Count (ms)() -> (millisecond timer value=w672:u32)
                        n282 = call "Wrapper_getSpectrum.vi"("Index"=0, "Wrapper"=w665) -> ("Spectrum Values"=w667:dbl[])  [unwired: 1 out]
                        n283 = Unbundle By Name(w674) -> ("Start time"=w673:i32)
                        n284 = Subtract(x=w672, y=w673) -> (x-y=w671:u32)
                        "Time during PD" <- w671
                        n285 = Bundle("Value"=w670, "Spectrum Values"=w667) -> (→"?":cluster{"Value":dbl[], "Spectrum Values":dbl[]})  [unwired: 1 in]
                        n286 = Build Array (concatenate)(w679, w671) -> (w680:u32[])
                        n287 = Build Array (concatenate)(w678, w667) -> (w675:dbl[][])
                      }
                      frame "Wait" {
                        n288 = Unbundle By Name(w693) -> ("Sample rate"=w694:dbl)
                        n289 = Multiply(x=1000.0, y="Slow sample time (s)") -> (x*y=w683:dbl)
                        n290 = Greater?(x=w684, y=w683) -> (0:w681:bool)
                        n291 = case shown="False" w681 {
                          tunnel: w694 -> [w695 _]
                          frame False {
                            n292 = Multiply(x=w695, y=1000.0) -> (x*y=w697:dbl)
                            n293 = Wait (ms)(milliseconds to wait=w697) -> ()  [unwired: 1 out]
                          }
                          frame True {
                            # "slow down read to measure slow decays\nwithout oversampling"
                            n294 = Wait (ms)(milliseconds to wait=u32 500) -> ()  [unwired: 1 out]
                          }
                        }
                      }
                    }
                  }
                  n295 = flat-sequence {
                    tunnel: [w624] -> w610
                    tunnel: [w623] -> w609
                    tunnel: w607 -> [w623]
                    tunnel: w608 -> [w622]
                    tunnel: w610 -> [w626]
                    tunnel: w609 -> [w625]
                    frame #0 {
                      # "Close spectrometers"
                      n296 = call "Wrapper_closeAllSpectrometers.vi"("Wrapper In"=w622) -> ("Wrapper Out"=w624:u32)
                    }
                    frame #1 {
                      # "Destroy \nwrapper \nand strobe"
                      n297 = call "ContinuousStrobe_Destroy.vi"("ContinuousStrobe"=w625) -> ()
                      n298 = call "Wrapper_Destroy.vi"("Wrapper"=w626) -> ()
                    }
                  }
                }
                frame True {
                  n299 = while {
                    shift-right: [w716] -> w699
                    shift-left: w706 -> [w717]
                    shift-right: [w709] -> _
                    shift-left: OSPEC-enum."Wait" -> [w718]
                    shift-right: [w715] -> w700
                    shift-left: w702 -> [w714]
                    shift-right: [w708] -> w701
                    shift-left: w704 -> [w713]
                    shift-right: [w712] -> _
                    shift-left: w705 -> [w711]
                    i -> [w710]
                    stop <- w707 stop-if-true
                    n300 = case shown="\"Wait\"" w718 {
                      tunnel: w717 -> [w720 _ w821]
                      tunnel: [w720 w729 w821] -> w716
                      tunnel: [w726 FALSE FALSE] -> w707
                      tunnel: [w728 w733 w819] -> w715
                      tunnel: w714 -> [w728 w737 w819]
                      tunnel: w710 -> [_ w740 _]
                      tunnel: w713 -> [w721 w736 w815]
                      tunnel: [w727 w731 w817] -> w712
                      tunnel: w711 -> [w727 w731 w817]
                      tunnel: [OSPEC-enum."Wait" OSPEC-enum."Check exit" OSPEC-enum."Read"] -> w709
                      tunnel: [w721 w734 w815] -> w708
                      frame "Check exit" {
                        n301 = Unbundle By Name(w727) -> ("V off time"=w722:dbl)
                        n302 = Multiply(x=w722, y=1000.0) -> (x*y=w723:dbl)
                        n303 = Greater Or Equal?(x=w720, y=w723) -> (x >= y?=w726:bool)
                      }
                      frame "Read", Default {
                        n304 = Unbundle By Name(w731) -> ("Start time"=w730:i32)
                        n305 = property on="Number of scans in kinetic cycle" class="DigNum (strict)"() -> ("Value"=w732:i32)  [unwired: 2 in, 2 out]
                        n306 = Tick Count (ms)() -> (millisecond timer value=w738:u32)
                        n307 = call "GetDetector.vi"() -> ("xpixels"=w739:i32)  [unwired: 4 in, 3 out]
                        n308 = Subtract(x=w738, y=w730) -> (x-y=w729:u32)
                        n309 = Equal?(x=w740, y=1.0) -> (x = y?=w735:bool)
                        n310 = stacked-sequence {
                          seq-local: [_ _ _ _ _ _ _ _ _ _ w774 _] -> [_ _ _ _ _ _ _ _ _ _ _ w794]
                          seq-local: [_ _ _ _ _ _ _ _ w759 _ _ _] -> [_ _ _ _ _ _ _ _ _ _ _ w792]
                          seq-local: [_ _ _ _ _ _ _ _ _ _ w773 _] -> [_ _ _ _ _ _ _ _ _ _ _ w793]
                          tunnel: [_ _ _ _ _ _ _ _ _ _ _ w787] -> w734
                          tunnel: [_ _ _ _ _ _ _ _ _ _ _ w788] -> w733
                          tunnel: w732 -> [_ _ _ _ _ w752 _ _ _ _ _ w786]
                          tunnel: w729 -> [_ _ _ _ _ _ _ _ _ _ _ w789]
                          tunnel: w729 -> [_ _ _ _ _ _ _ _ _ _ _ _]
                          tunnel: w739 -> [_ w745 _ _ _ _ _ _ _ _ _ _]
                          tunnel: w730 -> [_ _ _ _ _ _ _ _ w758 _ w772 _]
                          tunnel: w737 -> [_ _ _ _ _ _ _ _ _ _ _ w785]
                          tunnel: w736 -> [_ _ _ _ _ _ _ _ _ _ _ w784]
                          tunnel: w735 -> [_ _ _ _ _ _ _ _ _ _ _ w783]
                          frame #0 {
                            w744 = u16 3  # AcquisitionMode
                            n311 = call "SetAcquisitionMode.vi"("mode"=w744) -> ()  [unwired: 1 in, 2 out]
                          }
                          frame #1 {
                            w746 = u16 0  # ReadMode
                            n312 = property on="xpixels" class="DigNum (strict)"("Value"=w745) -> ()  [unwired: 2 in, 2 out]
                            n313 = call "SetReadMode.vi"("mode"=w746) -> ()  [unwired: 1 in, 2 out]
                          }
                          frame #2 {
                            n314 = call "SetTriggerMode.vi"("mode"=TriggerMode_mode_typedef."Internal") -> ()  [unwired: 1 in, 2 out]
                          }
                          frame #3 {
                            n315 = property on="Exposure time (s)" class="DigNum (strict)"() -> ("Value"=w748:dbl)  [unwired: 2 in, 2 out]
                            n316 = call "SetExposureTime.vi"("time"=w748) -> ()  [unwired: 1 in, 2 out]
                          }
                          frame #4 {
                            n317 = call "GetNumberVSSpeeds.vi"() -> ("number"=w751:i32)  [unwired: 3 in, 2 out]
                            n318 = Subtract(x=w751, y=1) -> (x-y=w749:i32)
                            n319 = call "SetVSSpeed.vi"("index"=w749) -> ()  [unwired: 1 in, 2 out]
                          }
                          frame #5 {
                            n320 = call "SetNumberKinetics.vi"("number"=w752) -> ()  [unwired: 1 in, 2 out]
                          }
                          frame #6 {
                            w755 = 0  # Auto Shutter
                            n321 = property on="Shutter open and close time" class="DigNum (strict)"() -> ("Value"=w753:i32)  [unwired: 2 in, 2 out]
                            n322 = property on="Shutter opens on TTL" class="Enum (strict)"() -> ("Value"=w754:T9)  [unwired: 2 in, 2 out]
                            n323 = call "SetShutter.vi"("type"=w754, "mode"=w755, "closingtime"=w753, "openingtime"=w753) -> ()  [unwired: 10 in, 2 out]
                          }
                          frame #7 {
                            # "Meybe delete the exposure time insupt here"
                            n324 = property on="Exposure time (s)" class="DigNum (strict)"() -> ("Value"=w757:dbl)  [unwired: 2 in, 2 out]
                            n325 = call "GetAcquisitionTimings.vi"("exposure input"=w757) -> ("exposure"=w756:sgl)  [unwired: 10 in, 4 out]
                            n326 = property on="Calculated exposure time" class="DigNum (strict)"("Value"=w756) -> ()  [unwired: 2 in, 2 out]
                          }
                          frame #8 {
                            n327 = flat-sequence {
                              tunnel: [w760] -> w759
                              tunnel: w758 -> [w761]
                              frame #0 {
                                n328 = Tick Count (ms)() -> (millisecond timer value=w762:u32)
                                n329 = Subtract(x=w762, y=w761) -> (x-y=w760:u32)
                                n330 = property on="Time before the start of current aquisition (ms)" class="DigNum (strict)"("Value"=w760) -> ()  [unwired: 2 in, 2 out]
                              }
                              frame #1 {
                                n331 = call "StartAcquisition.vi"() -> ("DLL error code"=w763:u32)  [unwired: 2 in, 1 out]
                                n332 = property on="Start Aquisition return code" class="DigNum (strict)"("Value"=w763) -> ()  [unwired: 2 in, 2 out]
                              }
                            }
                          }
                          frame #9 {
                            n333 = while {
                              stop <- w767 continue-if-true
                              w768 = u16 72  # DRV ACQUIRING
                              n334 = call "GetStatus.vi"() -> ("DLL error code"=w765:u32, "status"=w766:T19)  [unwired: 3 in, 1 out]
                              n335 = property on="Get status return code" class="DigNum (strict)"("Value"=w765) -> ()  [unwired: 2 in, 2 out]
                              n336 = Equal?(x=w766, y=w768) -> (x = y?=w767:bool)
                              n337 = property on="IDus not in read loop? (kinetic)" class="Bool (strict)"("Value"=FALSE ("IDus not in read loop? (kinetic)")) -> ()  [unwired: 2 in, 2 out]
                            }
                          }
                          frame #10 {
                            n338 = flat-sequence {
                              tunnel: [w775] -> w773
                              tunnel: w772 -> [w776]
                              tunnel: [w782] -> w774
                              tunnel: w771 -> [w779]
                              frame #0 {
                                n339 = Tick Count (ms)() -> (millisecond timer value=w777:u32)
                                n340 = Subtract(x=w777, y=w776) -> (x-y=w775:u32)
                                n341 = property on="Time  after the aquisition (before fetch data), (ms)" class="DigNum (strict)"("Value"=w775) -> ()  [unwired: 2 in, 2 out]
                              }
                              frame #1 {
                                n342 = call "GetAcquiredData.vi"("size"=w779) -> ("DLL error code"=w780:u32, "array"=w782:i32[])  [unwired: 2 in, 1 out]
                                n343 = Equal?(x=20002 ("DRV_SUCCESS"), y=w780) -> (x = y?=w778:bool)
                                n344 = property on="get aquired data return code" class="DigNum (strict)"("Value"=w780) -> ()  [unwired: 2 in, 2 out]
                                n345 = property on="Get aqisition ok? (kinetic mode)" class="Bool (strict)"("Value"=w778) -> ()  [unwired: 2 in, 2 out]
                              }
                            }
                            n346 = property on="Number of scans in kinetic cycle" class="DigNum (strict)"() -> ("Value"=w769:i32)  [unwired: 2 in, 2 out]
                            n347 = Multiply(x=1024.0, y=w769) -> (x*y=w771:dbl)
                          }
                          frame #11 {
                            n348 = Subtract(x=w793, y=w792) -> (x-y=w791:u32)
                            n349 = Divide(x=w791, y=w786) -> (x/y=w790:dbl)
                            n350 = for {
                              N: w786 -> [_]
                              tunnel: w794 -> [w808]
                              tunnel: w790 -> [w806]
                              tunnel: w789 -> [w804]
                              shift-right: [w802] -> w787
                              shift-left: w784 -> [w801]
                              shift-right: [w798] -> w788
                              shift-left: w785 -> [w799]
                              tunnel: w783 -> [_]
                              i -> [w796]
                              w803 = 1024 ("x")
                              n351 = Multiply(x=w796, y=w806) -> (x*y=w805:dbl)
                              n352 = Multiply(x=w803, y=w796) -> (x*y=w807:i32)
                              n353 = Add(x=w805, y=w804) -> (x+y=w800:dbl)
                              n354 = Array Subset(array=w808, index=w807, length=w803) -> (w795:i32[])
                              n355 = Equal To 0?(x=w796) -> (x = 0?=w797:bool)
                              n356 = case shown="True" w797 {
                                tunnel: w795 -> [_ w810]
                                frame False {
                                }
                                frame True {
                                n357 = for {
                                N: 1023 -> [_]
                                tunnel: [w813] -> w811 mode=indexing
                                i -> [w814]
                                n358 = Increment(x=w814) -> (x+1=w813:i32)
                                }
                                n359 = Bundle(w811, w810) -> (w809:cluster{i32[], i32[]})  [unwired: 1 in]
                                n360 = property class="XYGraph (strict)"("Value"=w809) -> ()  [unwired: 2 in, 2 out]
                                }
                              }
                              n361 = Build Array (concatenate)(w801, w795) -> (w802:dbl[][])
                              n362 = Build Array (concatenate)(w799, w800) -> (w798:dbl[])
                            }
                          }
                        }
                      }
                      frame "Wait" {
                        n363 = Unbundle By Name(w817) -> ("Sample rate"=w816:dbl)
                        n364 = Multiply(x=w816, y=1000.0) -> (x*y=w823:dbl)
                        n365 = Wait (ms)(milliseconds to wait=w823) -> ()  [unwired: 1 out]
                      }
                    }
                    n366 = case shown="True" w707 {
                      selector: w707 -> [_ w719]
                      frame False {
                      }
                      frame True {
                        n367 = property on="IDus not in read loop? (kinetic)" class="Bool (strict)"("Value"=w719) -> ()  [unwired: 2 in, 2 out]
                      }
                    }
                  }
                }
              }
              n368 = Bundle By Name(cluster=w569, "Time for spectrum measurment"=w583, "Time elapsed"=w584, "Spectrum"=w573) -> (w580:T11)
              n369 = Bundle By Name(cluster=w580, "Time for E measurment"=w582, "Potential array"=w581) -> (w575:T11)
            }
            frame "Read current and spectrum" {
              n370 = Unbundle By Name(w956) -> ("Time for spectrum measurment"=w970:i32[], "Start time"=w975:i32)
              n371 = Unbundle By Name(w956) -> ("Current array"=w969:dbl[])
              n372 = Unbundle By Name(w956) -> ("Time for I measurment"=w968:i32[], "Start time"=w974:i32)
              n373 = property on="V2 applied?" class="Bool (strict)"() -> ("Value"=w957:bool)  [unwired: 2 in, 2 out]
              n374 = case shown="False" w957 {
                tunnel: w956 -> [w991 w993]
                tunnel: [w990 w992] -> w955
                frame False {
                  n375 = Unbundle By Name(w991) -> ("V 1"=w990:dbl)
                }
                frame True {
                  n376 = Unbundle By Name(w993) -> ("V 2"=w992:dbl)
                }
              }
              n377 = local read "V (during measurment)"() -> (w976:dbl)
              n378 = Unbundle By Name(w956) -> ("V 1"=w977:dbl, "Spectrum"=w973:dbl[][])
              n379 = property on="Square wave?" class="Bool (strict)"() -> ("Value"=w962:bool)  [unwired: 2 in, 2 out]
              n380 = property on="V2 applied?" class="Bool (strict)"() -> ("Value"=w961:bool)  [unwired: 2 in, 2 out]
              n381 = property on="Use iDus?" class="Bool (strict)"() -> ("Value"=w967:bool)  [unwired: 2 in, 2 out]
              n382 = Equal?(x=w976, y=w977) -> (x = y?=w954:bool)
              n383 = And(x=w962, y=w961) -> (x .and. y?=w958:bool)
              n384 = Not(x=w958) -> (.not. x?=w960:bool)
              n385 = And(x=w954, y=w960) -> (x .and. y?=w959:bool)
              n386 = while {
                shift-right: [w1314] -> _
                shift-left: w956 -> [w1315]
                shift-right: [w1306] -> _
                shift-left: OSPEC-enum."Wait" -> [w1316]
                shift-right: [w1313] -> w980
                shift-left: w968 -> [w1312]
                shift-right: [w1307] -> w966
                shift-left: w969 -> [w1310]
                shift-right: [w1309] -> _
                shift-left: w974 -> [w1308]
                tunnel: w959 -> [w1305]
                shift-right: [w1303] -> w971
                shift-left: w972 -> [w1304]
                tunnel: w955 -> [w1299]
                i -> [w1311]
                stop <- w1300 stop-if-true
                n387 = case shown="\"Wait\"" w1316 {
                  tunnel: w1315 -> [w1330 w1361 w1471]
                  tunnel: [w1329 w1361 w1471] -> w1314
                  tunnel: [w1327 FALSE FALSE] -> w1301
                  tunnel: [w1332 w1369 w1469] -> w1313
                  tunnel: w1312 -> [w1332 w1370 w1469]
                  tunnel: w1311 -> [_ w1375 _]
                  tunnel: [w1324 w1374 w1467] -> w1307
                  tunnel: w1310 -> [w1324 w1373 w1467]
                  tunnel: [w1322 w1362 w1462] -> w1309
                  tunnel: w1308 -> [w1322 _ w1462]
                  tunnel: [OSPEC-enum."Wait" OSPEC-enum."Check exit" OSPEC-enum."Read"] -> w1306
                  tunnel: w1305 -> [_ w1364 _]
                  tunnel: w1304 -> [w1323 w1356 w1466]
                  tunnel: [w1323 w1359 w1466] -> w1303
                  tunnel: w1299 -> [_ w1355 _]
                  frame "Check exit" {
                    n388 = local read "V (during measurment)"() -> (w1326:dbl)
                    n389 = property on="Square wave?" class="Bool (strict)"() -> ("Value"=w1320:bool)  [unwired: 2 in, 2 out]
                    n390 = property on="V2 applied?" class="Bool (strict)"() -> ("Value"=w1321:bool)  [unwired: 2 in, 2 out]
                    n391 = Unbundle By Name(w1330) -> ("V 1"=w1331:dbl)
                    n392 = Equal?(x=w1331, y=w1326) -> (x = y?=w1328:bool)
                    n393 = And(x=w1320, y=w1321) -> (x .and. y?=w1319:bool)
                    n394 = case shown="True" w1328 {
                      tunnel: w1330 -> [w1338 w1342]
                      tunnel: [w1338 w1342] -> w1329
                      tunnel: [w1337 w1341] -> w1327
                      tunnel: w1322 -> [w1336 w1340]
                      tunnel: w1319 -> [_ w1339]
                      frame False {
                        n395 = Unbundle By Name(w1338) -> ("V2 time"=w1334:dbl)
                        n396 = Multiply(x=1000.0, y=w1334) -> (x*y=w1335:dbl)
                        n397 = Greater Or Equal?(x=w1336, y=w1335) -> (x >= y?=w1337:bool)
                      }
                      frame True {
                        n398 = case shown="False" w1339 {
                          tunnel: w1342 -> [w1345 w1354]
                          tunnel: [w1343 w1353] -> w1341
                          tunnel: w1340 -> [w1344 w1352]
                          frame False {
                            n399 = Unbundle By Name(w1345) -> ("V1 time"=w1348:dbl)
                            n400 = Multiply(x=w1348, y=1000.0) -> (x*y=w1347:dbl)
                            n401 = Greater Or Equal?(x=w1344, y=w1347) -> (x >= y?=w1343:bool)
                          }
                          frame True {
                            n402 = Unbundle By Name(w1354) -> ("V off time"=w1350:dbl)
                            n403 = Multiply(x=w1350, y=1000.0) -> (x*y=w1351:dbl)
                            n404 = Greater Or Equal?(x=w1352, y=w1351) -> (x >= y?=w1353:bool)
                          }
                        }
                      }
                    }
                  }
                  frame "Read", Default {
                    # "Building a 1d matrix of currents"
                    n405 = property on="Use autolab?" class="Bool (strict)"() -> ("Value"=w1357:bool)  [unwired: 2 in, 2 out]
                    n406 = case shown="True" w1357 {
                      tunnel: [w1379 w1387] -> w1368
                      tunnel: [w1378 w1388] -> w1359
                      tunnel: w1356 -> [w1377 w1386]
                      tunnel: w1355 -> [_ w1389]
                      tunnel: w1355 -> [_ w1383]
                      tunnel: w1356 -> [_ w1385]
                      tunnel: w1355 -> [_ w1384]
                      frame False {
                        n407 = flat-sequence {
                          tunnel: w1377 -> [w1381]
                          tunnel: [w1380] -> w1376
                          frame #0 {
                            n408 = call "IV getcurrent.vi"("error in (no error)"=w1381) -> ("error out"=w1380:errorcluster, "value out"=w1382:dbl)  [unwired: 8 in, 1 out]
                            n409 = call "Current ranging routine (SubVI).vi"("Current"=w1382) -> ()  [unwired: 11 in]
                          }
                        }
                        n410 = call "IV getcurrent.vi"("error in (no error)"=w1376) -> ("error out"=w1378:errorcluster, "value out"=w1379:dbl)  [unwired: 8 in, 1 out]
                      }
                      frame True {
                        n411 = disable-structure shown="Enabled" {
                          disable-tunnel: w1389 -> [w1407 _]
                          disable-tunnel: [w1401 w1427] -> w1388
                          disable-tunnel: [w1399 w1426] -> w1387
                          disable-tunnel: w1386 -> [w1394 _]
                          disable-tunnel: w1385 -> [w1393 w1442]
                          disable-tunnel: w1384 -> [w1390 _]
                          disable-tunnel: w1383 -> [_ w1445]
                          frame Disabled {
                            n412 = property on="Ei" class="Ref (strict)"() -> ("Value"=w1391:refnum<k24>)  [unwired: 2 in, 2 out]
                            n413 = disable-structure shown="Disabled" {
                              disable-tunnel: w1407 -> [w1419 _]
                              disable-tunnel: [w1418 _] -> _
                              disable-tunnel: w1394 -> [w1415 _]
                              disable-tunnel: w1391 -> [w1414 _]
                              frame Disabled {
                                w1412 = 2 items=["UltraHigh_Speed", "High_Speed", "High_Stability"] ("Bandwidth")
                                w1417 = 1 items=["Off", "On"] ("CellOnOff")
                                w1413 = 0 items=["Potentiostatic", "Galvanostatic"] ("Mode")
                                n414 = property on="CurrentRange" class="DigNum (strict)"() -> ("Value"=w1416:i32)  [unwired: 2 in, 2 out]
                                n415 = property class="EI"(reference=w1414, error in=w1415, "Bandwidth"=w1412, "CellOnOff"=w1417, "CurrentRange"=w1416, "Mode"=w1413, "Setpoint"=w1419) -> (error out=w1418:errorcluster)  [unwired: 1 out]
                                n416 = property on="Sampler 2" class="Ref (strict)"(error in=w1418) -> (error out=w1411:errorcluster, "Value"=w1408:refnum<k24>)  [unwired: 1 in, 1 out]
                                n417 = property class="EI"(reference=w1414, error in=w1418) -> (error out=w1409:errorcluster, "EiStatusSupportedFor"=w1410:string[])  [unwired: 1 out]
                                n418 = invoke class="Sampler" method="Sample"(reference=w1408, error in=w1411) -> ()  [unwired: 1 in, 3 out]
                                n419 = property on="EI status supported for" class="Arr (strict)"(error in=w1409, "Value"=w1410) -> ()  [unwired: 1 in, 2 out]
                              }
                              frame Enabled {
                              }
                            }
                            n420 = property class="EI"(reference=w1391, error in=w1393, "Setpoint"=w1390) -> (error out=w1392:errorcluster)  [unwired: 1 out]
                            n421 = property class="EI" props=["Bandwidth", "CurrentRange", "Mode", "Setpoint", "Current", "Potential"](reference=w1391, error in=w1392) -> (error out=w1395:errorcluster, "Bandwidth"=w1406:i32, "CurrentRange"=w1405:i32, "Mode"=w1404:i32, "Current"=w1398:dbl, "Potential"=w1397:dbl)  [unwired: 2 out]
                            n422 = property on="Bandwidth" class="DigNum (strict)"("Value"=w1406) -> ()  [unwired: 2 in, 2 out]
                            n423 = property on="CurrentRange" class="DigNum (strict)"("Value"=w1405) -> ()  [unwired: 2 in, 2 out]
                            n424 = property on="Mode" class="DigNum (strict)"("Value"=w1404) -> ()  [unwired: 2 in, 2 out]
                            n425 = flat-sequence {
                              tunnel: [w1423] -> w1403
                              tunnel: w1398 -> [w1422]
                              tunnel: w1397 -> [w1421]
                              tunnel: [w1420] -> w1396
                              tunnel: w1395 -> [w1420]
                              frame #0 {
                                n426 = call "Range_selector.vi"("potential"=w1421, "current"=w1422) -> ("range integer"=w1423:i32)  [unwired: 9 in]
                              }
                            }
                            n427 = property class="EI"(reference=w1391, error in=w1396) -> (error out=w1402:errorcluster, "Current"=w1399:dbl, "Potential"=→"POtential PD":dbl)  [unwired: 1 out]
                            "Current PD" <- w1399
                            n428 = property class="EI"(reference=w1391, error in=w1402, "CurrentRange"=w1403) -> (error out=w1401:errorcluster)  [unwired: 1 out]
                          }
                          frame Enabled {
                            w1429 = 0 items=["Potentiostatic", "Galvanostatic"] ("Mode")
                            w1430 = 1 items=["Off", "On"] ("CellOnOff")
                            w1431 = 1 items=["UltraHigh_Speed", "High_Speed", "High_Stability"] ("Bandwidth")
                            w1435 = 1 items=["Off", "On"] ("CellOnOff")
                            w1436 = 1 items=["UltraHigh_Speed", "High_Speed", "High_Stability"] ("Bandwidth")
                            w1437 = 0 items=["Potentiostatic", "Galvanostatic"] ("Mode")
                            w1446 = 0 items=["Potentiostatic", "Galvanostatic"] ("Mode")
                            w1448 = 1 items=["Off", "On"] ("CellOnOff")
                            w1449 = 1 items=["UltraHigh_Speed", "High_Speed", "High_Stability"] ("Bandwidth")
                            n429 = property on="Sampler 2" class="Ref (strict)"() -> ("Value"=w1433:refnum<k24>)  [unwired: 2 in, 2 out]
                            n430 = property on="CurrentRange" class="DigNum (strict)"() -> ("Value"=w1424:i32)  [unwired: 2 in, 2 out]
                            n431 = property on="Ei" class="Ref (strict)"() -> ("Value"=w1432:refnum<k24>)  [unwired: 2 in, 2 out]
                            n432 = call "EI (A).vi"("Sampler"=w1433, "Ei"=w1432, "CellOnOff"=w1448, "Setpoint"=w1445, "Bandwidth"=w1449, "CurrentRange"=w1424, "Mode"=w1446, "error in (no error)"=w1442, "Disable Sampler"=FALSE) -> ("Cell"=w1443:bool, "Bandwidth"=w1444:i32, "error out"=w1441:errorcluster)  [unwired: 5 in, 11 out]
                            n433 = property on="Bandwidth" class="DigNum (strict)"("Value"=w1444) -> ()  [unwired: 2 in, 2 out]
                            n434 = property on="Cell on?" class="Bool (strict)"("Value"=w1443) -> ()  [unwired: 2 in, 2 out]
                            n435 = call "Sampler.vi"("error in (no error)"=w1442, "Sampler"=w1433) -> ("error out"=w1439:errorcluster)  [unwired: 7 in, 2 out]
                            n436 = Merge Errors(w1439, w1441) -> (w1440:errorcluster)
                            n437 = call "EI (A).vi"("Sampler"=w1433, "Ei"=w1432, "CellOnOff"=w1435, "Bandwidth"=w1436, "Mode"=w1437, "error in (no error)"=w1440, "Disable Sampler"=FALSE) -> ("Potential"=w1434:dbl, "Current"=w1426:dbl, "error out"=w1428:errorcluster)  [unwired: 7 in, 11 out]
                            "Current during PD" <- w1426
                            n438 = property on="Voltage" class="DigNum (strict)"("Value"=w1434) -> ()  [unwired: 2 in, 2 out]
                            n439 = property on="current" class="DigNum (strict)"("Value"=w1426) -> ()  [unwired: 2 in, 2 out]
                            n440 = call "Range_selector.vi"("potential"=w1434, "current"=w1426) -> ("range integer"=w1425:i32)  [unwired: 9 in]
                            n441 = call "EI (A).vi"("Sampler"=w1433, "Ei"=w1432, "CellOnOff"=w1430, "Bandwidth"=w1431, "Mode"=w1429, "error in (no error)"=w1428) -> ("error out"=w1427:errorcluster)  [unwired: 8 in, 13 out]
                            n442 = property on="CurrentRange" class="DigNum (strict)"("Value"=w1425) -> ()  [unwired: 2 in, 2 out]
                          }
                        }
                      }
                    }
                    n443 = Unbundle By Name(w1361) -> ("Start time"=w1360:i32)
                    n444 = Tick Count (ms)() -> (millisecond timer value=w1358:u32)
                    n445 = Subtract(x=w1358, y=w1360) -> (x-y=w1371:u32)
                    n446 = Equal?(x=1, y=w1375) -> (x = y?=w1365:bool)
                    n447 = And(x=w1364, y=w1365) -> (x .and. y?=w1363:bool)
                    n448 = case shown="True" w1363 {
                      tunnel: [w1451 w1455] -> w1369
                      tunnel: w1370 -> [w1452 w1453]
                      tunnel: w1371 -> [w1450 w1454]
                      tunnel: [w1450 w1454] -> w1362
                      frame False {
                        n449 = Build Array (concatenate)(w1452, w1450) -> (w1451:u32[])
                      }
                      frame True {
                        n450 = Build Array (concatenate)(w1453, w1454) -> (w1455:u32[])
                      }
                    }
                    n451 = case shown="True" w1363 {
                      tunnel: [w1457 w1459] -> w1374
                      tunnel: w1373 -> [w1458 _]
                      tunnel: w1368 -> [w1456 w1460]
                      frame False {
                        # "Intensity thereafter"
                        n452 = Build Array (concatenate)(w1458, w1456) -> (w1457:dbl[])
                      }
                      frame True {
                        n453 = Build Array(w1460) -> (w1459:dbl[])
                      }
                    }
                  }
                  frame "Wait" {
                    w1464 = 1000.0 ("y")
                    n454 = Unbundle By Name(w1471) -> ("Sample rate"=w1472:dbl)
                    n455 = property on="Slow sample time (s)" class="DigNum (strict)"() -> ("Value"=w1465:dbl)  [unwired: 2 in, 2 out]
                    n456 = Multiply(x=w1464, y=w1465) -> (x*y=w1463:dbl)
                    n457 = Greater?(x=w1462, y=w1463) -> (0:w1461:bool)
                    n458 = case shown="False" w1461 {
                      tunnel: w1464 -> [_ w1474]
                      tunnel: w1472 -> [_ w1473]
                      frame False {
                      }
                      frame True {
                        n459 = Multiply(x=w1473, y=w1474) -> (x*y=w1475:dbl)
                        n460 = Wait (ms)(milliseconds to wait=w1475) -> ()  [unwired: 1 out]
                      }
                    }
                  }
                }
                n461 = property on="Use iDus?" class="Bool (strict)"() -> ("Value"=w1298:bool)  [unwired: 2 in, 2 out]
                n462 = case shown="False" w1298 {
                  tunnel: [TRUE ("Value") w1318] -> w1302
                  frame False {
                  }
                  frame True {
                    n463 = property on="IDus not in read loop? (kinetic)" class="Bool (strict)"() -> ("Value"=w1318:bool)  [unwired: 2 in, 2 out]
                  }
                }
                n464 = And(x=w1302, y=w1301) -> (x .and. y?=w1300:bool)
              }
              n465 = case shown="True" w967 {
                tunnel: [w1007 w1120] -> w983
                tunnel: [w1006 w1122] -> w982
                tunnel: [w1001 w1119] -> w981
                tunnel: w975 -> [w1005 w1121]
                tunnel: w959 -> [w1004 w1125]
                tunnel: w973 -> [w1003 w1126]
                tunnel: w970 -> [w1002 w1124]
                tunnel: w956 -> [w995 w1123]
                tunnel: w954 -> [w994 w1118]
                tunnel: w958 -> [_ w1117]
                frame False {
                  n466 = case shown="True" w994 {
                    tunnel: w995 -> [_ w1017]
                    tunnel: [w1009 w1014] -> w1000
                    tunnel: [w1010 w1012] -> w998
                    tunnel: [w1011 w1013] -> w996
                    frame False {
                      n467 = property on="Wrapper Out" class="DigNum (strict)"() -> ("Value"=w1011:u32)  [unwired: 2 in, 2 out]
                      n468 = property on="ContinuousStrobe Out" class="DigNum (strict)"() -> ("Value"=w1010:u32)  [unwired: 2 in, 2 out]
                      n469 = property on="WL Values" class="Arr (strict)"() -> ("Value"=w1009:dbl[])  [unwired: 2 in, 2 out]
                    }
                    frame True {
                      n470 = Unbundle By Name(w1017) -> ("Continous strobe delay"=w1015:i32, "Integration time"=w1016:i32)
                      n471 = call "OSPEC-Open-Ocean.vi"("Integration Time"=w1016, "delay"=w1015) -> ("WL Values"=w1014:dbl[], "Wrapper Out"=w1013:u32, "ContinuousStrobe Out"=w1012:u32)  [unwired: 7 in]
                      "ContinuousStrobe Out" <- w1012
                      "Wrapper Out" <- w1013
                      "WL Values" <- w1014
                    }
                  }
                  n472 = while {
                    shift-right: [w1042] -> _
                    shift-left: w995 -> [w1043]
                    shift-right: [w1034] -> _
                    shift-left: OSPEC-enum."Wait" -> [w1044]
                    shift-right: [w1040] -> w1001
                    shift-left: w1002 -> [w1039]
                    shift-right: [w1032] -> w1006
                    shift-left: w1003 -> [w1038]
                    shift-right: [w1037] -> w1007
                    shift-left: w1005 -> [w1036]
                    tunnel: w1004 -> [w1033]
                    tunnel: w1000 -> [w1031]
                    tunnel: [w1030] -> w999
                    tunnel: w996 -> [w1027]
                    tunnel: w998 -> [w1028]
                    tunnel: [w1029] -> w997
                    i -> [w1035]
                    stop <- w1041 stop-if-true
                    n473 = case shown="\"Wait\"" w1044 {
                      tunnel: w1043 -> [w1053 w1074 w1112]
                      tunnel: [w1052 w1074 w1112] -> w1042
                      tunnel: [w1050 FALSE FALSE] -> w1041
                      tunnel: [w1054 w1088 w1110] -> w1040
                      tunnel: w1039 -> [w1054 w1087 w1110]
                      tunnel: w1035 -> [_ w1082 _]
                      tunnel: [w1047 w1076 w1108] -> w1032
                      tunnel: w1038 -> [w1047 w1086 w1108]
                      tunnel: [w1051 w1077 w1105] -> w1037
                      tunnel: w1036 -> [w1051 _ w1105]
                      tunnel: [OSPEC-enum."Wait" OSPEC-enum."Check exit" OSPEC-enum."Read"] -> w1034
                      tunnel: w1033 -> [w1048 w1081 _]
                      tunnel: w1031 -> [_ w1067 _]
                      tunnel: [w1046 w1071 w1107] -> w1030
                      tunnel: w1028 -> [w1046 w1071 w1107]
                      tunnel: w1027 -> [w1045 w1070 w1106]
                      tunnel: [w1045 w1070 w1106] -> w1029
                      frame "Check exit" {
                        n474 = case shown="False" w1048 {
                          tunnel: w1053 -> [w1060 w1066]
                          tunnel: [w1060 w1066] -> w1052
                          tunnel: w1051 -> [w1058 w1064]
                          tunnel: [w1059 w1065] -> w1050
                          frame False {
                            n475 = Unbundle By Name(w1060) -> ("V2 time"=w1057:dbl)
                            n476 = Multiply(x=w1057, y=1000.0) -> (x*y=w1055:dbl)
                            n477 = Greater Or Equal?(x=w1058, y=w1055) -> (x >= y?=w1059:bool)
                          }
                          frame True {
                            n478 = Unbundle By Name(w1066) -> ("V1 time"=w1063:dbl)
                            n479 = Multiply(x=w1063, y=1000.0) -> (x*y=w1061:dbl)
                            n480 = Greater Or Equal?(x=w1064, y=w1061) -> (x >= y?=w1065:bool)
                          }
                        }
                      }
                      frame "Read", Default {
                        # "Check here to see if DIM t + 1 and DIM WL match"
                        n481 = Tick Count (ms)() -> (millisecond timer value=w1072:u32)
                        n482 = call "Wrapper_getSpectrum.vi"("Index"=0, "Wrapper"=w1070) -> ("Spectrum Values"=w1068:dbl[])  [unwired: 1 out]
                        n483 = Unbundle By Name(w1074) -> ("Start time"=w1073:i32)
                        n484 = Subtract(x=w1072, y=w1073) -> (x-y=w1078:u32)
                        n485 = Bundle("WL Values"=w1067, "Spectrum Values"=w1068) -> (→"?":T5)  [unwired: 1 in]
                        n486 = Equal?(x=w1082, y=1.0) -> (x = y?=w1080:bool)
                        n487 = And(x=w1081, y=w1080) -> (x .and. y?=w1079:bool)
                        n488 = case shown="False" w1079 {
                          tunnel: [w1091 w1092] -> w1076
                          tunnel: w1086 -> [w1090 _]
                          tunnel: w1068 -> [w1089 w1094]
                          tunnel: w1067 -> [_ w1093]
                          frame False {
                            # "Intensity thereafter"
                            n489 = Build Array (concatenate)(w1090, w1089) -> (w1091:dbl[][])
                          }
                          frame True {
                            n490 = Build Array(w1093, w1094) -> (w1092:dbl[][])
                          }
                        }
                        n491 = case shown="True" w1079 {
                          tunnel: [w1097 w1100] -> w1088
                          tunnel: w1087 -> [w1096 w1099]
                          tunnel: w1078 -> [w1095 w1098]
                          tunnel: [w1095 w1098] -> w1077
                          frame False {
                            n492 = Build Array (concatenate)(w1096, w1095) -> (w1097:u32[])
                          }
                          frame True {
                            n493 = Build Array (concatenate)(w1099, w1098) -> (w1100:u32[])
                          }
                        }
                      }
                      frame "Wait" {
                        n494 = Unbundle By Name(w1112) -> ("Sample rate"=w1113:dbl)
                        n495 = property on="Slow sample time (s)" class="DigNum (strict)"() -> ("Value"=w1102:dbl)  [unwired: 2 in, 2 out]
                        n496 = Multiply(x=w1102, y=1000.0) -> (x*y=w1101:dbl)
                        n497 = Greater?(x=w1105, y=w1101) -> (0:w1104:bool)
                        n498 = case shown="True" w1104 {
                          tunnel: w1113 -> [_ w1114]
                          frame False {
                          }
                          frame True {
                            n499 = Multiply(x=w1114, y=1000.0) -> (x*y=w1116:dbl)
                            n500 = Wait (ms)(milliseconds to wait=w1116) -> ()  [unwired: 1 out]
                          }
                        }
                      }
                    }
                  }
                  n501 = disable-structure shown="Disabled" {
                    disable-tunnel: w999 -> [w1019 _]
                    disable-tunnel: w997 -> [w1018 _]
                    frame Disabled {
                      n502 = flat-sequence {
                        tunnel: [w1024] -> w1021
                        tunnel: [w1023] -> w1020
                        tunnel: w1019 -> [w1023]
                        tunnel: w1018 -> [w1022]
                        tunnel: w1021 -> [w1026]
                        tunnel: w1020 -> [w1025]
                        frame #0 {
                          # "Close spectrometers"
                          n503 = call "Wrapper_closeAllSpectrometers.vi"("Wrapper In"=w1022) -> ("Wrapper Out"=w1024:u32)
                        }
                        frame #1 {
                          # "Destroy \nwrapper \nand strobe"
                          n504 = call "ContinuousStrobe_Destroy.vi"("ContinuousStrobe"=w1025) -> ()
                          n505 = call "Wrapper_Destroy.vi"("Wrapper"=w1026) -> ()
                        }
                      }
                    }
                    frame Enabled {
                    }
                  }
                }
                frame True {
                  n506 = while {
                    shift-right: [w1140] -> w1120
                    shift-left: w1121 -> [w1141]
                    shift-right: [w1133] -> _
                    shift-left: OSPEC-enum."Wait" -> [w1142]
                    shift-right: [w1139] -> w1119
                    shift-left: w1124 -> [w1138]
                    shift-right: [w1131] -> w1122
                    shift-left: w1126 -> [w1137]
                    shift-right: [w1136] -> _
                    shift-left: w1123 -> [w1135]
                    tunnel: w1125 -> [w1132]
                    tunnel: w1118 -> [w1129]
                    tunnel: w1117 -> [w1128]
                    i -> [w1134]
                    stop <- w1130 stop-if-true
                    n507 = case shown="\"Wait\"" w1142 {
                      tunnel: w1141 -> [w1151 _ w1285]
                      tunnel: [w1150 w1178 w1285] -> w1140
                      tunnel: [w1148 FALSE FALSE] -> w1130
                      tunnel: [w1152 w1179 w1293] -> w1139
                      tunnel: w1138 -> [w1152 w1184 w1293]
                      tunnel: w1134 -> [_ w1188 _]
                      tunnel: w1137 -> [w1146 w1182 w1289]
                      tunnel: [w1149 w1177 w1291] -> w1136
                      tunnel: w1135 -> [w1149 w1177 w1291]
                      tunnel: [OSPEC-enum."Wait" OSPEC-enum."Check exit" OSPEC-enum."Read"] -> w1133
                      tunnel: w1132 -> [_ w1183 _]
                      tunnel: [w1146 w1180 w1289] -> w1131
                      tunnel: w1129 -> [w1145 _ _]
                      tunnel: w1128 -> [w1144 _ _]
                      frame "Check exit" {
                        n508 = case shown="True" w1145 {
                          tunnel: w1151 -> [w1154 w1163]
                          tunnel: [w1154 w1162] -> w1150
                          tunnel: w1149 -> [w1153 w1161]
                          tunnel: [w1155 w1160] -> w1148
                          tunnel: w1144 -> [_ w1159]
                          frame False {
                            n509 = Unbundle By Name(w1153) -> ("V2 time"=w1156:dbl)
                            n510 = Multiply(x=w1156, y=1000.0) -> (x*y=w1157:dbl)
                            n511 = Greater Or Equal?(x=w1154, y=w1157) -> (x >= y?=w1155:bool)
                          }
                          frame True {
                            n512 = case shown="False" w1159 {
                              tunnel: w1163 -> [w1165 w1170]
                              tunnel: [w1165 w1170] -> w1162
                              tunnel: w1161 -> [w1164 w1171]
                              tunnel: [w1169 w1175] -> w1160
                              frame False {
                                n513 = Unbundle By Name(w1164) -> ("V1 time"=w1166:dbl)
                                n514 = Multiply(x=w1166, y=1000.0) -> (x*y=w1167:dbl)
                                n515 = Greater Or Equal?(x=w1165, y=w1167) -> (x >= y?=w1169:bool)
                              }
                              frame True {
                                n516 = Unbundle By Name(w1171) -> ("V off time"=w1172:dbl)
                                n517 = Multiply(x=w1172, y=1000.0) -> (x*y=w1173:dbl)
                                n518 = Greater Or Equal?(x=w1170, y=w1173) -> (x >= y?=w1175:bool)
                              }
                            }
                          }
                        }
                      }
                      frame "Read", Default {
                        n519 = Unbundle By Name(w1177) -> ("Start time"=w1176:i32)
                        n520 = property on="Number of scans in kinetic cycle" class="DigNum (strict)"() -> ("Value"=w1187:i32)  [unwired: 2 in, 2 out]
                        n521 = Tick Count (ms)() -> (millisecond timer value=w1185:u32)
                        n522 = Subtract(x=w1185, y=w1176) -> (x-y=w1178:u32)
                        n523 = call "GetDetector.vi"() -> ("xpixels"=w1186:i32)  [unwired: 4 in, 3 out]
                        n524 = Equal?(x=w1188, y=1.0) -> (x = y?=w1181:bool)
                        n525 = stacked-sequence {
                          seq-local: [_ _ _ _ _ _ _ _ _ _ w1222 _] -> [_ _ _ _ _ _ _ _ _ _ _ w1243]
                          seq-local: [_ _ _ _ _ _ _ _ w1207 _ _ _] -> [_ _ _ _ _ _ _ _ _ _ _ w1241]
                          seq-local: [_ _ _ _ _ _ _ _ _ _ w1221 _] -> [_ _ _ _ _ _ _ _ _ _ _ w1242]
                          tunnel: [_ _ _ _ _ _ _ _ _ _ _ w1236] -> w1180
                          tunnel: [_ _ _ _ _ _ _ _ _ _ _ w1237] -> w1179
                          tunnel: w1187 -> [_ _ _ _ _ w1200 _ _ _ _ w1218 w1235]
                          tunnel: w1178 -> [_ _ _ _ _ _ _ _ _ _ _ w1238]
                          tunnel: w1186 -> [_ w1193 _ _ _ _ _ _ _ _ _ _]
                          tunnel: w1176 -> [_ _ _ _ _ _ _ _ w1206 _ w1220 _]
                          tunnel: w1184 -> [_ _ _ _ _ _ _ _ _ _ _ w1234]
                          tunnel: w1183 -> [_ _ _ _ _ _ _ _ _ _ _ w1233]
                          tunnel: w1182 -> [_ _ _ _ _ _ _ _ _ _ _ w1232]
                          tunnel: w1181 -> [_ _ _ _ _ _ _ _ _ _ _ w1231]
                          frame #0 {
                            w1192 = u16 3  # AcquisitionMode
                            n526 = call "SetAcquisitionMode.vi"("mode"=w1192) -> ()  [unwired: 1 in, 2 out]
                          }
                          frame #1 {
                            w1194 = u16 0  # ReadMode
                            n527 = property on="xpixels" class="DigNum (strict)"("Value"=w1193) -> ()  [unwired: 2 in, 2 out]
                            n528 = call "SetReadMode.vi"("mode"=w1194) -> ()  [unwired: 1 in, 2 out]
                          }
                          frame #2 {
                            n529 = call "SetTriggerMode.vi"("mode"=TriggerMode_mode_typedef."Internal") -> ()  [unwired: 1 in, 2 out]
                          }
                          frame #3 {
                            n530 = property on="Exposure time (s)" class="DigNum (strict)"() -> ("Value"=w1196:dbl)  [unwired: 2 in, 2 out]
                            n531 = call "SetExposureTime.vi"("time"=w1196) -> ()  [unwired: 1 in, 2 out]
                          }
                          frame #4 {
                            n532 = call "GetNumberVSSpeeds.vi"() -> ("number"=w1199:i32)  [unwired: 3 in, 2 out]
                            n533 = Subtract(x=w1199, y=1) -> (x-y=w1197:i32)
                            n534 = call "SetVSSpeed.vi"("index"=w1197) -> ()  [unwired: 1 in, 2 out]
                          }
                          frame #5 {
                            n535 = call "SetNumberKinetics.vi"("number"=w1200) -> ()  [unwired: 1 in, 2 out]
                          }
                          frame #6 {
                            w1203 = 0  # Auto Shutter
                            n536 = call "SetShutter.vi"("type"="Shutter opens on TTL", "mode"=w1203, "closingtime"="Shutter open and close time", "openingtime"="Shutter open and close time") -> ()  [unwired: 10 in, 2 out]
                          }
                          frame #7 {
                            # "Meybe delete the exposure time insupt here"
                            n537 = property on="Exposure time (s)" class="DigNum (strict)"() -> ("Value"=w1204:dbl)  [unwired: 2 in, 2 out]
                            n538 = call "GetAcquisitionTimings.vi"("exposure input"=w1204) -> ("exposure"=w1205:sgl)  [unwired: 10 in, 4 out]
                            n539 = property on="Calculated exposure time" class="DigNum (strict)"("Value"=w1205) -> ()  [unwired: 2 in, 2 out]
                          }
                          frame #8 {
                            n540 = flat-sequence {
                              tunnel: [w1209] -> w1207
                              tunnel: w1206 -> [w1208]
                              frame #0 {
                                n541 = Tick Count (ms)() -> (millisecond timer value=w1210:u32)
                                n542 = Subtract(x=w1210, y=w1208) -> (x-y=w1209:u32)
                                "Time before the start of current aquisition (ms)" <- w1209
                              }
                              frame #1 {
                                n543 = call "StartAcquisition.vi"() -> ("DLL error code"=w1211:u32)  [unwired: 2 in, 1 out]
                                n544 = property on="Start Aquisition return code" class="DigNum (strict)"("Value"=w1211) -> ()  [unwired: 2 in, 2 out]
                              }
                            }
                          }
                          frame #9 {
                            n545 = while {
                              stop <- w1215 continue-if-true
                              w1216 = u16 72  # DRV ACQUIRING
                              n546 = call "GetStatus.vi"() -> ("DLL error code"=w1213:u32, "status"=w1214:T19)  [unwired: 3 in, 1 out]
                              n547 = property on="Get status return code" class="DigNum (strict)"("Value"=w1213) -> ()  [unwired: 2 in, 2 out]
                              n548 = Equal?(x=w1214, y=w1216) -> (x = y?=w1215:bool)
                              "IDus not in read loop? (kinetic)" <- FALSE
                            }
                          }
                          frame #10 {
                            n549 = flat-sequence {
                              tunnel: [w1223] -> w1221
                              tunnel: w1220 -> [w1224]
                              tunnel: [w1230] -> w1222
                              tunnel: w1219 -> [w1226]
                              frame #0 {
                                n550 = Tick Count (ms)() -> (millisecond timer value=w1225:u32)
                                n551 = Subtract(x=w1225, y=w1224) -> (x-y=w1223:u32)
                                "Time  after the aquisition (before fetch data), (ms)" <- w1223
                              }
                              frame #1 {
                                n552 = call "GetAcquiredData.vi"("size"=w1226) -> ("DLL error code"=w1227:u32, "array"=w1230:i32[])  [unwired: 2 in, 1 out]
                                n553 = Equal?(x=20002 ("DRV_SUCCESS"), y=w1227) -> (x = y?=→"Get aqisition ok? (kinetic mode)":bool)
                                n554 = property on="get aquired data return code" class="DigNum (strict)"("Value"=w1227) -> ()  [unwired: 2 in, 2 out]
                              }
                            }
                            n555 = Multiply(x=1024, y=w1218) -> (x*y=w1219:i32)
                          }
                          frame #11 {
                            n556 = Subtract(x=w1242, y=w1241) -> (x-y=w1240:u32)
                            n557 = Divide(x=w1240, y=w1235) -> (x/y=w1239:dbl)
                            n558 = for {
                              N: w1235 -> [_]
                              tunnel: w1243 -> [w1261]
                              tunnel: w1239 -> [w1259]
                              tunnel: w1238 -> [w1256]
                              shift-right: [w1254] -> w1236
                              shift-left: w1232 -> [w1253]
                              shift-right: [w1246] -> w1237
                              shift-left: w1234 -> [w1251]
                              tunnel: w1233 -> [w1249]
                              tunnel: w1231 -> [w1247]
                              i -> [w1245]
                              w1255 = 1024 ("x")
                              n559 = Equal To 0?(x=w1245) -> (x = 0?=w1244:bool)
                              n560 = Multiply(x=w1245, y=w1259) -> (x*y=w1258:dbl)
                              n561 = Multiply(x=w1255, y=w1245) -> (x*y=w1260:i32)
                              n562 = Add(x=w1258, y=w1256) -> (x+y=w1252:dbl)
                              n563 = Array Subset(array=w1261, index=w1260, length=w1255) -> (w1257:i32[])
                              n564 = And(x=w1244, y=w1247) -> (x .and. y?=w1248:bool)
                              n565 = And(x=w1249, y=w1248) -> (x .and. y?=w1250:bool)
                              n566 = case shown="False" w1250 {
                                tunnel: w1257 -> [w1262 w1275]
                                tunnel: [w1267 w1278] -> w1254
                                tunnel: w1253 -> [w1268 _]
                                tunnel: w1252 -> [w1265 w1280]
                                tunnel: [w1264 w1279] -> w1246
                                tunnel: w1251 -> [w1266 _]
                                tunnel: w1244 -> [w1263 _]
                                frame False {
                                n567 = case shown="True" w1263 {
                                tunnel: w1262 -> [_ w1271]
                                frame False {
                                }
                                frame True {
                                n568 = for {
                                N: 1023 -> [_]
                                tunnel: [w1273] -> _ mode=indexing
                                tunnel: [w1273] -> w1270 mode=indexing
                                i -> [w1274]
                                n569 = Increment(x=w1274) -> (x+1=w1273:i32)
                                }
                                n570 = Bundle(w1270, w1271) -> (w1269:cluster{i32[], i32[]})  [unwired: 1 in]
                                n571 = property class="XYGraph (strict)"("Value"=w1269) -> ()  [unwired: 2 in, 2 out]
                                }
                                }
                                n572 = Build Array (concatenate)(w1268, w1262) -> (w1267:dbl[][])
                                n573 = Build Array (concatenate)(w1266, w1265) -> (w1264:dbl[])
                                }
                                frame True {
                                n574 = for {
                                N: 1023 -> [_]
                                tunnel: [w1282] -> w1276 mode=indexing
                                i -> [w1283]
                                n575 = Increment(x=w1283) -> (x+1=w1282:i32)
                                }
                                n576 = Bundle(w1276, w1275) -> (w1277:cluster{i32[], i32[]})  [unwired: 1 in]
                                n577 = Build Array(w1280) -> (w1279:dbl[])
                                n578 = Build Array(w1276, w1275) -> (w1278:i32[][])
                                n579 = property class="XYGraph (strict)"("Value"=w1277) -> ()  [unwired: 2 in, 2 out]
                                }
                              }
                            }
                          }
                        }
                      }
                      frame "Wait" {
                        w1288 = 1000.0 ("y")
                        n580 = Unbundle By Name(w1291) -> ("Sample rate"=w1290:dbl)
                        n581 = property on="Slow sample time (s)" class="DigNum (strict)"() -> ("Value"=w1287:dbl)  [unwired: 2 in, 2 out]
                        n582 = Multiply(x=w1288, y=w1287) -> (x*y=w1286:dbl)
                        n583 = Greater?(x=w1285, y=w1286) -> (0:w1284:bool)
                        n584 = case shown="True" w1284 {
                          tunnel: w1290 -> [_ w1296]
                          tunnel: w1288 -> [_ w1295]
                          frame False {
                          }
                          frame True {
                            n585 = Multiply(x=w1296, y=w1295) -> (x*y=w1297:dbl)
                            n586 = Wait (ms)(milliseconds to wait=w1297) -> ()  [unwired: 1 out]
                          }
                        }
                      }
                    }
                    n587 = case shown="True" w1130 {
                      frame False {
                      }
                      frame True {
                        n588 = property on="IDus not in read loop? (kinetic)" class="Bool (strict)"("Value"=TRUE ("IDus not in read loop? (kinetic)")) -> ()  [unwired: 2 in, 2 out]
                      }
                    }
                  }
                }
              }
              n589 = Bundle By Name(cluster=w956, "Time for spectrum measurment"=w981, "Time elapsed"=w983, "Spectrum"=w982) -> (w978:T11)
              n590 = Bundle By Name(cluster=w978, "Time for I measurment"=w980, "Current array"=w966) -> (w979:T11)
              n591 = local read "V (during measurment)"() -> (w985:dbl)
              n592 = property on="V2 applied?" class="Bool (strict)"() -> ("Value"=w965:bool)  [unwired: 2 in, 2 out]
              n593 = Unbundle By Name(w978) -> ("V 1"=w986:dbl)
              n594 = Equal?(x=w986, y=w985) -> (x = y?=w987:bool)
              n595 = And(x=w965, y="Square wave?") -> (x .and. y?=w964:bool)
              n596 = case shown="False" w987 {
                tunnel: [w1477 w1481] -> w988
                tunnel: w964 -> [_ w1480]
                tunnel: "Square wave?" -> [w1476 _]
                frame False {
                  n597 = case shown="False" w1476 {
                    tunnel: [OSSPEC."Read Potential and spectrum" OSSPEC."Apply V1"] -> w1477
                    frame False {
                    }
                    frame True {
                    }
                  }
                }
                frame True {
                  n598 = case shown="False" w1480 {
                    tunnel: [OSSPEC."Apply V2" OSSPEC."End measurment"] -> w1481
                    frame False {
                    }
                    frame True {
                    }
                  }
                }
              }
            }
            frame "Reinitialise Cell" {
              # "this state is no longer used as it adds a 1-300 ms delay before the spectrum is measured as the mode is shifted"
              n599 = flat-sequence {
                tunnel: w1490 -> [w1494]
                tunnel: [w1493] -> w1485
                tunnel: w1485 -> [w1497]
                tunnel: [w1496] -> w1484
                tunnel: [w1498] -> w1489
                tunnel: w1484 -> [w1498]
                frame #0 {
                  n600 = To Long Integer(number=T17."IStat4EL" ("Configuration")) -> (32bit integer=w1492:i32)
                  n601 = call "IV setconnectionmode.vi"("error in (no error)"=w1494, "value"=w1492) -> ("error out"=w1493:errorcluster)  [unwired: 7 in, 2 out]
                }
                frame #1 {
                  n602 = call "IV setcurrent.vi"("error in (no error)"=w1497, "value"=0.0) -> ("error out"=w1496:errorcluster)  [unwired: 7 in, 2 out]
                }
                frame #2 {
                }
              }
              n603 = Unbundle By Name(w1486) -> ()  [unwired: 3 out]
            }
            frame "Apply V1" {
              n604 = property on="Use autolab?" class="Bool (strict)"() -> ("Value"=w1502:bool)  [unwired: 2 in, 2 out]
              n605 = property on="Potential  During PD" class="WFChart (strict)"("History Data"=dbl[] []) -> ()  [unwired: 2 in, 2 out]
              n606 = property on="Current during PD" class="WFChart (strict)"("History Data"=dbl[] []) -> ()  [unwired: 2 in, 2 out]
              n607 = flat-sequence {
                tunnel: w1510 -> [w1516]
                tunnel: w1509 -> [w1515]
                tunnel: [w1514] -> w1504
                tunnel: [w1513] -> w1503
                tunnel: w1502 -> [w1512]
                tunnel: [w1511] -> w1501
                tunnel: w1510 -> [w1557]
                tunnel: w1504 -> [w1555]
                tunnel: [w1556] -> w1506
                tunnel: [w1551] -> w1505
                tunnel: w1503 -> [w1550]
                tunnel: w1502 -> [w1549]
                tunnel: w1501 -> [w1548]
                frame #0 {
                  n608 = case shown="True" w1512 {
                    tunnel: w1516 -> [w1522 w1539]
                    tunnel: w1515 -> [w1521 _]
                    tunnel: [w1520 w1531] -> w1514
                    tunnel: [w1518 w1538] -> w1513
                    tunnel: [refnum<k24> refnum ("Value") w1535] -> w1511
                    frame False {
                      n609 = Unbundle By Name(w1522) -> ("V 1"=w1520:dbl)
                      n610 = Absolute Value(x=w1520) -> (abs(x)=w1524:dbl)
                      n611 = local write "V (during measurment)"(w1520) -> ()
                      n612 = Greater?(x=w1524, y=3.0) -> (0:w1523:bool)
                      n613 = case shown="False" w1523 {
                        tunnel: [w1525 w1527] -> w1518
                        tunnel: w1521 -> [w1525 w1526]
                        frame False {
                        }
                        frame True {
                          # "abort if E >3 V"
                          n614 = call "IV setcellon.vi"("error in (no error)"=w1526, "cellon"=0) -> ("error out"=w1529:errorcluster)  [unwired: 7 in, 2 out]
                          n615 = call "IV close.vi"("error in (no error)"=w1529) -> ("error out"=w1527:errorcluster)  [unwired: 9 in, 1 out]
                          n616 = call "Display Message to User3"("error in (no error)"=w1527) -> ("OK"=w1530:bool)  [unwired: 9 in, 1 out]
                          n617 = Stop(stop? (T)=w1530) -> ()
                        }
                      }
                    }
                    frame True {
                      w1545 = 1 items=["Off", "On"] ("CellOnOff")
                      n618 = property on="Ei" class="Ref (strict)"() -> ("Value"=w1535:refnum<k24>)  [unwired: 2 in, 2 out]
                      n619 = property on="Sampler 2" class="Ref (strict)"() -> ("Value"=w1541:refnum<k24>)  [unwired: 2 in, 2 out]
                      n620 = property class="EI" props=["EiStatusSupportedFor"](reference=w1535) -> (error out=w1537:errorcluster)  [unwired: 1 in, 2 out]
                      n621 = property class="EI" props=["Bandwidth", "CurrentRange", "Mode", "Potential", "Current"](reference=w1535) -> (error out=w1543:errorcluster, "Potential"=w1547:dbl, "Current"=w1546:dbl)  [unwired: 1 in, 4 out]
                      n622 = invoke class="Sampler" method="Sample"(reference=w1541) -> (error out=w1536:errorcluster)  [unwired: 2 in, 2 out]
                      n623 = Unbundle By Name(w1539) -> ("V 1"=w1531:dbl)
                      n624 = call "Range_selector.vi"("potential"=w1547, "current"=w1546) -> ("range integer"=w1544:i32)  [unwired: 9 in]
                      n625 = property class="EI"(reference=w1535, error in=w1543, "CellOnOff"=w1545, "CurrentRange"=w1544) -> (error out=w1542:errorcluster)  [unwired: 1 out]
                      n626 = call "P_Stat_Status1.vi"("error in (no error)"=w1542, ".NET Refnum in"=w1535) -> ("error out"=w1540:errorcluster, "PotentialOverload"=w1532:bool, "CurrentOverload"=w1534:bool, "Cell"=w1533:bool)  [unwired: 3 in, 3 out]
                      n627 = Merge Errors(w1540, w1537, w1536) -> (w1538:errorcluster)
                      n628 = property on="V (during measurment)" class="DigNum (strict)"("Value"=w1531) -> ()  [unwired: 2 in, 2 out]
                      n629 = property on="Cell on?" class="Bool (strict)"("Value"=w1533) -> ()  [unwired: 2 in, 2 out]
                      n630 = property on="PotentialOverload" class="Bool (strict)"("Value"=w1532) -> ()  [unwired: 2 in, 2 out]
                      n631 = property on="CurrentOverload" class="Bool (strict)"("Value"=w1534) -> ()  [unwired: 2 in, 2 out]
                    }
                  }
                }
                frame #1 {
                  n632 = property on="Square wave?" class="Bool (strict)"() -> ("Value"=w1553:bool)  [unwired: 2 in, 2 out]
                  n633 = property on="V2 applied?" class="Bool (strict)"() -> ("Value"=w1554:bool)  [unwired: 2 in, 2 out]
                  n634 = case shown="True" w1549 {
                    tunnel: w1555 -> [w1560 w1563]
                    tunnel: [w1559 w1562] -> w1551
                    tunnel: w1550 -> [w1558 w1564]
                    tunnel: w1548 -> [_ w1561]
                    frame False {
                      n635 = call "IV setpotential.vi"("error in (no error)"=w1558, "value"=w1560) -> ("error out"=w1559:errorcluster)  [unwired: 7 in, 2 out]
                    }
                    frame True {
                      n636 = property class="EI"(reference=w1561, error in=w1564, "Setpoint"=w1563) -> (error out=w1562:errorcluster)  [unwired: 1 out]
                    }
                  }
                  n637 = And(x=w1553, y=w1554) -> (x .and. y?=w1552:bool)
                  n638 = case shown="False" w1552 {
                    tunnel: w1557 -> [w1568 w1569]
                    tunnel: [w1567 w1569] -> w1556
                    frame False {
                      n639 = Tick Count (ms)() -> (millisecond timer value=w1565:u32)
                      n640 = Bundle By Name(cluster=w1568, "Start time"=w1565, "Time elapsed"=0) -> (w1567:T11)
                    }
                    frame True {
                    }
                  }
                }
              }
            }
            frame "Apply V2" {
              n641 = Tick Count (ms)() -> (millisecond timer value=w1577:u32)
              n642 = flat-sequence {
                tunnel: w1572 -> [w1590]
                tunnel: [w1591] -> w1583
                tunnel: w1582 -> [w1589]
                tunnel: [w1584] -> w1579
                tunnel: [w1588] -> w1578
                tunnel: w1577 -> [w1588]
                tunnel: w1572 -> [w1587]
                tunnel: [w1586] -> w1571
                tunnel: [w1585] -> w1570
                tunnel: w1583 -> [w1627]
                tunnel: w1579 -> [w1626]
                tunnel: w1578 -> [w1625]
                tunnel: [w1625] -> w1575
                tunnel: [w1624] -> w1573
                tunnel: w1571 -> [w1622]
                tunnel: w1570 -> [w1621]
                frame #0 {
                  n643 = property on="Use autolab?" class="Bool (strict)"() -> ("Value"=w1586:bool)  [unwired: 2 in, 2 out]
                  n644 = Unbundle By Name(w1590) -> ("V 2"=w1584:dbl)
                  n645 = Absolute Value(x=w1584) -> (abs(x)=w1594:dbl)
                  n646 = Greater?(x=w1594, y=3.0) -> (0:w1592:bool)
                  n647 = local write "V (during measurment)"(w1584) -> ()
                  n648 = case shown="True" w1586 {
                    tunnel: w1592 -> [w1598 _]
                    tunnel: [w1597 w1612] -> w1591
                    tunnel: w1589 -> [w1596 _]
                    tunnel: w1587 -> [_ _]
                    tunnel: [refnum<k24> refnum ("Value") w1611] -> w1585
                    tunnel: w1584 -> [_ w1609]
                    frame False {
                      n649 = case shown="True" w1598 {
                        tunnel: [w1599 w1601] -> w1597
                        tunnel: w1596 -> [w1599 w1600]
                        frame False {
                        }
                        frame True {
                          # "abort if E >3 V"
                          n650 = call "IV setcellon.vi"("error in (no error)"=w1600, "cellon"=0) -> ("error out"=w1603:errorcluster)  [unwired: 7 in, 2 out]
                          n651 = call "IV close.vi"("error in (no error)"=w1603) -> ("error out"=w1601:errorcluster)  [unwired: 9 in, 1 out]
                          n652 = call "Display Message to User4"("error in (no error)"=w1601) -> ("OK"=w1604:bool)  [unwired: 9 in, 1 out]
                          n653 = Stop(stop? (T)=w1604) -> ()
                        }
                      }
                    }
                    frame True {
                      w1605 = -2 items=["CR07_1A"=0, "CR06_10A"=1, "CR01_100A"=2, "CR00_1000A"=3, "CR05_20A"=20, "CR04_40A"=40, "CR03_50A"=60, "CR02_80A"=80, "CR19_1pA"=-12, "CR18_10pA"=-11, "CR17_100pA"=-10, "CR16_1nA"=-9, "CR15_10nA"=-8, "CR14_100nA"=-7, "CR13_1uA"=-6, "CR12_10uA"=-5, "CR11_100uA"=-4, "CR10_1mA"=-3, "CR09_10mA"=-2, "CR08_100mA"=-1] ("CurrentRange")
                      w1618 = 1 items=["Off", "On"] ("CellOnOff")
                      n654 = property on="Ei" class="Ref (strict)"() -> ("Value"=w1611:refnum<k24>)  [unwired: 2 in, 2 out]
                      n655 = property on="Sampler 2" class="Ref (strict)"() -> ("Value"=w1613:refnum<k24>)  [unwired: 2 in, 2 out]
                      n656 = property class="EI"(reference=w1611) -> (error out=w1610:errorcluster, "EiStatusSupportedFor"=w1608:string[])  [unwired: 1 in, 1 out]
                      n657 = property class="EI" props=["Bandwidth", "CurrentRange", "Mode", "Potential", "Current"](reference=w1611) -> (error out=w1617:errorcluster, "Potential"=w1620:dbl, "Current"=w1619:dbl)  [unwired: 1 in, 4 out]
                      n658 = invoke class="Sampler" method="Sample"(reference=w1613) -> (error out=w1614:errorcluster)  [unwired: 2 in, 2 out]
                      n659 = call "Range_selector.vi"("potential"=w1620, "current"=w1619) -> ()  [unwired: 9 in, 1 out]
                      n660 = property on="EI status supported for" class="Arr (strict)"("Value"=w1608) -> ()  [unwired: 2 in, 2 out]
                      n661 = property class="EI"(reference=w1611, error in=w1617, "CellOnOff"=w1618, "CurrentRange"=w1605, "Setpoint"=w1609) -> (error out=w1616:errorcluster)  [unwired: 1 out]
                      n662 = property on="CurrentRange" class="DigNum (strict)"("Value"=w1605) -> ()  [unwired: 2 in, 2 out]
                      n663 = call "P_Stat_Status1.vi"("error in (no error)"=w1616, ".NET Refnum in"=w1611) -> ("error out"=w1615:errorcluster, "PotentialOverload"=w1606:bool, "CurrentOverload"=w1607:bool)  [unwired: 3 in, 4 out]
                      n664 = property on="CurrentOverload" class="Bool (strict)"("Value"=w1607) -> ()  [unwired: 2 in, 2 out]
                      n665 = Merge Errors(w1615, w1610, w1614) -> (w1612:errorcluster)
                      n666 = property on="PotentialOverload" class="Bool (strict)"("Value"=w1606) -> ()  [unwired: 2 in, 2 out]
                    }
                  }
                }
                frame #1 {
                  n667 = case shown="False" w1622 {
                    tunnel: w1627 -> [w1630 w1633]
                    tunnel: w1626 -> [w1629 w1631]
                    tunnel: [w1628 w1632] -> w1624
                    tunnel: w1621 -> [_ w1634]
                    frame False {
                      n668 = call "IV setpotential.vi"("error in (no error)"=w1630, "value"=w1629) -> ("error out"=w1628:errorcluster)  [unwired: 7 in, 2 out]
                    }
                    frame True {
                      n669 = property class="EI"(reference=w1634, error in=w1633, "Setpoint"=w1631) -> (error out=w1632:errorcluster)  [unwired: 1 out]
                    }
                  }
                  "V2 applied?" <- TRUE ("V2 applied")
                }
              }
              n670 = Tick Count (ms)() -> (millisecond timer value=w1574:u32)
              n671 = Subtract(x=w1574, y=w1575) -> (x-y=→"Time taken to apply V2":u32)
              n672 = Unbundle By Name(w1572) -> ()  [unwired: 3 out]
            }
            frame "End measurment" {
              w1645 = ext 0.00099999999999999999996
              w1662 = TRUE
              n673 = Unbundle By Name(w1635) -> ("Time for spectrum measurment"=w1641:i32[], "Spectrum"=w1658:dbl[][])
              n674 = Unbundle By Name(w1635) -> ("Current array"=w1652:dbl[], "Time for I measurment"=w1647:i32[])
              n675 = Unbundle By Name(w1635) -> ("Time for E measurment"=w1644:i32[], "Potential array"=w1653:dbl[])
              n676 = Multiply(x=w1641, y=ext 0.00099999999999999999996) -> (x*y=w1640:ext[])
              n677 = Multiply(x=w1647, y=w1645) -> (x*y=w1646:ext[])
              n678 = Multiply(x=w1645, y=w1644) -> (x*y=w1643:ext[])
              n679 = Build Array(w1646, w1652) -> (w1651:ext[][])
              n680 = Build Array(w1643, w1653) -> (w1649:ext[][])
              n681 = Insert Into Array(array=w1640, index=0, new element=0 ("new element/subarray")) -> (w1656:ext[])
              n682 = Transpose 2D Array(2D array=w1651) -> (transposed array=w1650:ext[][])
              n683 = Transpose 2D Array(2D array=w1649) -> (transposed array=w1648:ext[][])
              n684 = Insert Into Array(array=w1658, index (col)=0 ("disabled index (col)"), new element=w1656) -> (w1655:dbl[][])  [unwired: 1 in]
              n685 = call "Write-OSP-J-t.vi"("Init cluster"=w1635, "Array"=w1650) -> ()  [unwired: 10 in]
              n686 = call "Write-OSP-E-t.vi"("Init cluster"=w1635, "Array"=w1648) -> ()  [unwired: 10 in]
              n687 = Transpose 2D Array(2D array=w1655) -> (transposed array=w1654:dbl[][])
              n688 = call "Write-OSP-SP.vi"("Init cluster"=w1635, "Array"=w1654) -> ()  [unwired: 10 in]
              n689 = property on="T reached?" class="Bool (strict)"("Value"=FALSE ("T reached?")) -> ()  [unwired: 2 in, 2 out]
              n690 = Unbundle By Name(w1635) -> ("Default\n potential"=w1637:dbl)
              n691 = property on="Use autolab?" class="Bool (strict)"() -> ("Value"=w1638:bool)  [unwired: 2 in, 2 out]
              n692 = case shown="True" w1638 {
                tunnel: w1637 -> [w1666 w1682]
                tunnel: w1663 -> [w1665 w1681]
                tunnel: [w1664 w1680] -> w1661
                frame False {
                  n693 = flat-sequence {
                    tunnel: w1665 -> [w1670]
                    tunnel: [w1669] -> w1668
                    tunnel: w1666 -> [w1675]
                    tunnel: w1668 -> [w1674]
                    tunnel: [w1673] -> w1667
                    tunnel: w1667 -> [w1677]
                    tunnel: [w1676] -> w1664
                    frame #0 {
                      n694 = To Long Integer(number=T17."EStat4EL" ("Configuration")) -> (32bit integer=w1672:i32)
                      n695 = call "IV setconnectionmode.vi"("error in (no error)"=w1670, "value"=w1672) -> ("error out"=w1669:errorcluster)  [unwired: 7 in, 2 out]
                    }
                    frame #1 {
                      n696 = call "IV setpotential.vi"("error in (no error)"=w1674, "value"=w1675) -> ("error out"=w1673:errorcluster)  [unwired: 7 in, 2 out]
                    }
                    frame #2 {
                      n697 = call "IV getcurrent.vi"("error in (no error)"=w1677) -> ("error out"=w1676:errorcluster, "value out"=w1678:dbl)  [unwired: 8 in, 1 out]
                      n698 = call "Current ranging routine (SubVI).vi"("Current"=w1678) -> ()  [unwired: 11 in]
                    }
                  }
                }
                frame True {
                  w1687 = 0 items=["Off", "On"] ("CellOnOff")
                  n699 = property on="Ei" class="Ref (strict)"() -> ("Value"=w1679:refnum<k24>)  [unwired: 2 in, 2 out]
                  n700 = disable-structure shown="Enabled" {
                    disable-tunnel: [w1707 _] -> w1685
                    disable-tunnel: [w1706 _] -> w1684
                    disable-tunnel: [w1705 -3 ("range integer")] -> w1683
                    disable-tunnel: w1682 -> [w1703 _]
                    disable-tunnel: w1681 -> [w1701 _]
                    disable-tunnel: w1679 -> [w1696 _]
                    frame Disabled {
                      w1702 = -2 items=["CR07_1A"=0, "CR06_10A"=1, "CR01_100A"=2, "CR00_1000A"=3, "CR05_20A"=20, "CR04_40A"=40, "CR03_50A"=60, "CR02_80A"=80, "CR19_1pA"=-12, "CR18_10pA"=-11, "CR17_100pA"=-10, "CR16_1nA"=-9, "CR15_10nA"=-8, "CR14_100nA"=-7, "CR13_1uA"=-6, "CR12_10uA"=-5, "CR11_100uA"=-4, "CR10_1mA"=-3, "CR09_10mA"=-2, "CR08_100mA"=-1] ("CurrentRange")
                      w1704 = 0 items=["Potentiostatic", "Galvanostatic"] ("Mode")
                      n701 = property class="EI"(reference=w1696, error in=w1701, "Setpoint"=w1703, "Mode"=w1704, "CurrentRange"=w1702) -> (error out=w1698:errorcluster)  [unwired: 1 out]
                      n702 = property on="Sampler 2" class="Ref (strict)"() -> ("Value"=w1697:refnum<k24>)  [unwired: 2 in, 2 out]
                      n703 = property class="EI"(reference=w1696, error in=w1698) -> ("Current"=w1699:dbl, "Potential"=w1700:dbl)  [unwired: 2 out]
                      n704 = property class="EI" props=["EiStatusSupportedFor"](reference=w1696) -> (error out=w1707:errorcluster)  [unwired: 1 in, 2 out]
                      n705 = invoke class="Sampler" method="Sample"(reference=w1697) -> (error out=w1706:errorcluster)  [unwired: 2 in, 2 out]
                      n706 = flat-sequence {
                        tunnel: [w1711] -> w1705
                        tunnel: w1700 -> [w1710]
                        tunnel: w1699 -> [w1709]
                        frame #0 {
                          n707 = Wait (ms)(milliseconds to wait=u32 50) -> ()  [unwired: 1 out]
                        }
                        frame #1 {
                          n708 = call "Range_selector.vi"("potential"=w1710, "current"=w1709) -> ("range integer"=w1711:i32)  [unwired: 9 in]
                        }
                      }
                    }
                    frame Enabled {
                    }
                  }
                  n709 = property class="EI"(reference=w1679, "CellOnOff"=w1687, "CurrentRange"=w1683) -> (error out=w1686:errorcluster)  [unwired: 1 in, 1 out]
                  n710 = disable-structure shown="Enabled" {
                    disable-tunnel: w1686 -> [w1695 _]
                    disable-tunnel: w1685 -> [w1693 _]
                    disable-tunnel: w1684 -> [w1692 _]
                    disable-tunnel: [w1691 _] -> w1680
                    disable-tunnel: w1679 -> [w1690 _]
                    frame Disabled {
                      n711 = call "P_Stat_Status1.vi"("error in (no error)"=w1695, ".NET Refnum in"=w1690) -> ("error out"=w1694:errorcluster, "PotentialOverload"=w1689:bool, "CurrentOverload"=w1688:bool)  [unwired: 3 in, 4 out]
                      n712 = property on="CurrentOverload" class="Bool (strict)"("Value"=w1688) -> ()  [unwired: 2 in, 2 out]
                      n713 = Merge Errors(w1694, w1693, w1692) -> (w1691:errorcluster)
                      n714 = property on="PotentialOverload" class="Bool (strict)"("Value"=w1689) -> ()  [unwired: 2 in, 2 out]
                    }
                    frame Enabled {
                    }
                  }
                }
              }
              "PD ENDED\nEXIT MEASURMENT" <- w1662
            }
          }
        }
        n715 = property on="PD ENDED\nEXIT MEASURMENT" class="Bool (strict)"() -> ("Value"=w535:bool)  [unwired: 2 in, 2 out]
        n716 = case shown="True" w535 {
          tunnel: [State."Wait for Event" ("f") State."Exit" ("f")] -> w544
          frame False {
          }
          frame True {
          }
        }
      }
      frame "Initialse and cool iDus" {
        # "Also re-intialise constants"
        n717 = Unbundle By Name(w1714) -> ("Return detector to \nroom T"=w1717:bool)
        n718 = case shown="False" w1717 {
          tunnel: [State."Wait for Event" ("f") State."Wait for Event" ("f")] -> w1716
          frame False {
            w1726 = 20002  # DRV_SUCCESS
            n719 = stacked-sequence {
              seq-local: [_ _ _ _ _ _ w1792] -> [_ _ _ _ _ _ _]
              seq-local: [_ _ _ _ _ _ w1793] -> [_ _ _ _ _ _ _]
              tunnel: w1726 -> [w1782 _ _ _ _ _ _]
              tunnel: [w1781 _ _ _ _ _ _] -> w1725
              tunnel: [_ _ _ _ _ _ w1792] -> _
              tunnel: [_ _ _ _ _ _ w1793] -> w1720
              frame #0 {
                n720 = call "Initialize.vi"("directory (\"\")"="" ("directory (\"\")")) -> ("DLL error code"=w1784:u32)  [unwired: 1 in, 1 out]
                "Init. return code" <- w1784
                n721 = Equal?(x=w1782, y=w1784) -> (x = y?=w1781:bool)
              }
              frame #1 {
                n722 = Wait (ms)(milliseconds to wait=u32 2000) -> ()  [unwired: 1 out]
              }
              frame #2 {
                w1786 = u16 0  # ReadMode
                n723 = call "SetReadMode.vi"("mode"=w1786) -> ()  [unwired: 1 in, 2 out]
              }
              frame #3 {
                w1787 = u16 1  # AcquisitionMode
                n724 = call "SetAcquisitionMode.vi"("mode"=w1787) -> ()  [unwired: 1 in, 2 out]
              }
              frame #4 {
                w1788 = 0
                n725 = call "SetHSSpeed.vi"("index"=w1788, "type"=w1788) -> ()  [unwired: 2 in, 2 out]
              }
              frame #5 {
                n726 = call "GetNumberVSSpeeds.vi"() -> ("number"=w1791:i32)  [unwired: 3 in, 2 out]
                n727 = Subtract(x=w1791, y=1) -> (x-y=w1789:i32)
                n728 = call "SetVSSpeed.vi"("index"=w1789) -> ()  [unwired: 1 in, 2 out]
              }
              frame #6 {
                n729 = call "GetDetector.vi"() -> ("ypixels"=w1792:i32, "xpixels"=w1793:i32)  [unwired: 4 in, 2 out]
                "xpixels" <- w1793
                "ypixels" <- w1792
              }
            }
            n730 = flat-sequence {
              tunnel: w1725 -> [w1777]
              tunnel: [w1776] -> w1724
              frame #0 {
                n731 = case shown="False" w1777 {
                  selector: w1777 -> [w1779 w1780]
                  tunnel: [w1778 w1780] -> w1776
                  frame False {
                    n732 = Not(x=w1779) -> (.not. x?=w1778:bool)
                    n733 = call "Display Message to User5"() -> ()  [unwired: 10 in, 2 out]
                    n734 = Stop(stop? (T)=w1778) -> ()
                  }
                  frame True {
                  }
                }
              }
            }
            n735 = flat-sequence {
              tunnel: w1724 -> [w1733]
              tunnel: [w1731] -> w1721
              tunnel: w1720 -> [w1731]
              tunnel: [w1730] -> _
              frame #0 {
                w1734 = 36  # DRV_TEMP_STABILIZED
                w1735 = 20002  # DRV_SUCCESS
                # "set T ok?"
                # "timings ok?"
                n736 = stacked-sequence {
                  seq-local: [_ _ w1738 _ _ _] -> [_ _ _ _ _ _]
                  seq-local: [_ _ _ w1746 _ _] -> [_ _ _ _ w1750 w1751]
                  tunnel: w1735 -> [_ _ w1740 w1749 _ _]
                  tunnel: "Temperature\n(degrees C)" -> [_ _ _ w1747 _ _]
                  tunnel: w1734 -> [_ _ _ _ _ w1752]
                  tunnel: w1733 -> [_ _ w1739 _ _ _]
                  tunnel: [_ _ _ _ _ w1751] -> w1730
                  frame #0 {
                    n737 = call "SetTriggerMode.vi"("mode"=TriggerMode_mode_typedef."Internal") -> ()  [unwired: 1 in, 2 out]
                  }
                  frame #1 {
                    n738 = property on="Exposure time (s)" class="DigNum (strict)"() -> ("Value"=w1737:dbl)  [unwired: 2 in, 2 out]
                    n739 = call "SetExposureTime.vi"("time"=w1737) -> ()  [unwired: 1 in, 2 out]
                  }
                  frame #2 {
                    n740 = case shown="True" w1739 {
                      tunnel: w1740 -> [_ w1744]
                      tunnel: [FALSE w1745] -> w1738
                      frame False {
                      }
                      frame True {
                        n741 = call "GetAcquisitionTimings.vi"() -> ("exposure"=→"Calculated exposure time":sgl, "DLL error code"=w1743:u32)  [unwired: 11 in, 3 out]
                        "Check timings return code" <- w1743
                        n742 = Equal?(x=w1744, y=w1743) -> (x = y?=w1745:bool)
                      }
                    }
                  }
                  frame #3 {
                    n743 = call "SetTemperature.vi"("temperature"=w1747) -> ("DLL error code"=w1748:u32)  [unwired: 1 in, 1 out]
                    "Set temprature\nreturn code" <- w1748
                    n744 = Equal?(x=w1749, y=w1748) -> (x = y?=w1746:bool)
                  }
                  frame #4 {
                    n745 = case shown="True" w1750 {
                      frame False {
                      }
                      frame True {
                        n746 = call "CoolerON.vi"() -> ()  [unwired: 2 in, 2 out]
                      }
                    }
                  }
                  frame #5 {
                    n747 = case shown="True" w1751 {
                      tunnel: w1752 -> [_ w1753]
                      frame False {
                      }
                      frame True {
                        n748 = while {
                          tunnel: w1753 -> [w1757]
                          stop <- w1754 continue-if-true
                          n749 = Wait Until Next ms Multiple(millisecond multiple=u32 500) -> ()  [unwired: 1 out]
                          n750 = call "GetTemperature.vi"() -> ("status"=w1755:T19, "temperature"=→"Curent Temp":i32)  [unwired: 4 in, 2 out]
                          n751 = Not Equal?(x=w1757, y=w1755) -> (x != y?=w1754:bool)
                        }
                      }
                    }
                  }
                }
              }
            }
            n752 = for {
              N: 1023 -> [_]
              tunnel: [w1727] -> w1718 mode=indexing
              i -> [w1729]
              n753 = Add(x=1, y=w1729) -> (x+y=w1727:i32)
            }
            n754 = stacked-sequence {
              seq-local: [w1760 _ _] -> [_ w1765 _]
              tunnel: TRUE -> [w1759 _ _]
              tunnel: w1721 -> [_ _ w1774]
              tunnel: w1718 -> [_ _ w1772]
              frame #0 {
                n755 = case shown="True" w1759 {
                  tunnel: [FALSE w1764] -> w1760
                  frame False {
                  }
                  frame True {
                    w1762 = 20002  # DRV_SUCCESS
                    n756 = call "StartAcquisition.vi"() -> ("DLL error code"=w1763:u32)  [unwired: 2 in, 1 out]
                    "Start Aquisition return code" <- w1763
                    n757 = Equal?(x=w1762, y=w1763) -> (x = y?=w1764:bool)
                  }
                }
              }
              frame #1 {
                n758 = case shown="True" w1765 {
                  frame False {
                  }
                  frame True {
                    n759 = while {
                      stop <- w1768 continue-if-true
                      w1767 = u16 72  # DRV ACQUIRING
                      n760 = call "GetStatus.vi"() -> ("status"=w1766:T19)  [unwired: 3 in, 2 out]
                      n761 = Wait Until Next ms Multiple(millisecond multiple=u32 50) -> ()  [unwired: 1 out]
                      n762 = property on="Get status return code" class="DigNum (strict)"("Value"=w1766) -> ()  [unwired: 2 in, 2 out]
                      n763 = Equal?(x=w1766, y=w1767) -> (x = y?=w1768:bool)
                    }
                  }
                }
              }
              frame #2 {
                n764 = call "GetAcquiredData.vi"("size"=w1774) -> ("DLL error code"=→"get aquired data return code":u32, "array"=w1771:i32[])  [unwired: 2 in, 1 out]
                n765 = Bundle(w1772, "array"=w1771) -> (→"?":cluster{i32[], "array":i32[]})  [unwired: 1 in]
                "T reached?" <- TRUE ("T reached?")
              }
            }
          }
          frame True {
            n766 = property on="T reached?" class="Bool (strict)"("Value"=FALSE ("T reached?")) -> ()  [unwired: 2 in, 2 out]
            n767 = stacked-sequence {
              frame #0 {
                n768 = call "CoolerOFF.vi"() -> ("DLL error code"=→"Cooler Off return code":u32)  [unwired: 2 in, 1 out]
              }
              frame #1 {
                n769 = while {
                  stop <- w1799 continue-if-true
                  n770 = call "GetTemperature.vi"() -> ("temperature"=w1797:i32)  [unwired: 4 in, 3 out]
                  n771 = property on="Curent Temp" class="DigNum (strict)"("Value"=w1797) -> ()  [unwired: 2 in, 2 out]
                  n772 = Less?(x=w1797, y=i16 0) -> (x < y?=w1799:bool)
                  n773 = Wait Until Next ms Multiple(millisecond multiple=u32 500) -> ()  [unwired: 1 out]
                }
              }
              frame #2 {
                n774 = call "ShutDown.vi"() -> ()  [unwired: 2 in, 2 out]
                "Shut down sequence run?" <- TRUE ("Shut down complete?")
              }
            }
          }
        }
      }
    }
    n775 = property on="Use autolab?" class="Bool (strict)"() -> ("Value"=w4:bool)  [unwired: 2 in, 2 out]
    n776 = Equal To 0?(x=w22) -> (x = 0?=w30:bool)
    n777 = case shown="True" w4 {
      tunnel: w31 -> [w47 w83]
      tunnel: w30 -> [w46 _]
      tunnel: [w45 w83] -> w24
      tunnel: [w42 FALSE] -> w20
      frame False {
        n778 = case shown="False" w46 {
          tunnel: w47 -> [w56 w82]
          tunnel: [w55 w80] -> w45
          tunnel: [w50 w74] -> w39
          tunnel: [w51 w75] -> w43
          tunnel: [w53 w81] -> w41
          tunnel: [w49 w73] -> w40
          tunnel: [w52 w76] -> w44
          frame False {
            n779 = call "IV getcellstatus.vi"() -> ("devcellstatus out"=w66:i32)  [unwired: 9 in, 2 out]
            n780 = call "Bitget 8-bits test.vi"("x"=w66) -> ("c"=w62:dbl, "e"=w64:dbl, "f"=w63:dbl, "h"=w65:dbl)  [unwired: 19 in, 4 out]
            n781 = Greater?(x=w62, y=0.0) -> (0:w68:bool)
            n782 = Greater?(x=w64, y=0.0) -> (0:w69:bool)
            n783 = Greater?(x=w63, y=0.0) -> (0:w70:bool)
            n784 = Greater?(x=w65, y=0.0) -> (0:w48:bool)
            n785 = And(x=w66, y=256) -> (x .and. y?=w67:i32)
            n786 = Equal?(x=w67, y=256) -> (x = y?=w71:bool)
            n787 = Bundle By Name(cluster=w56, "I overload"=w68, "Aninput1 overload"=w69, "E overload"=w70, "Cell of button pressed"=w48, "Cell on"=w71) -> (w55:T11)
            n788 = Unbundle By Name(w55) -> ("I overload"=w53:bool, "Aninput1 overload"=w52:bool, "E overload"=w51:bool, "Cell of button pressed"=w50:bool, "Cell on"=w49:bool)
          }
          frame True {
            w72 = FALSE
            # "After closing the driver reset the indicators"
            n789 = property class="XYGraph (strict)"("Value"=cluster{dbl[], dbl[]} {[], []} ("XY Graph")) -> ()  [unwired: 2 in, 2 out]
            n790 = property on="Potentiostat Status" class="Str"("Value"="" ("Device Status indicator")) -> ()  [unwired: 2 in, 2 out]
            n791 = property on="Device serial number" class="Str"("Value"="" ("Device serial number")) -> ()  [unwired: 2 in, 2 out]
            n792 = Bundle By Name(cluster=w82, "I overload"=w72, "Aninput1 overload"=w72, "E overload"=w72, "Cell of button pressed"=w72, "Cell on"=w72) -> (w80:T11)
            n793 = Unbundle By Name(w80) -> ("I overload"=w81:bool, "Aninput1 overload"=w76:bool, "E overload"=w75:bool, "Cell of button pressed"=w74:bool, "Cell on"=w73:bool)
          }
        }
        "I_overload" <- w41
        "Aninput1_overload" <- w44
        "E_overload" <- w43
        "cell-off button pressed" <- w39
        "cell on" <- w40
        n794 = Or(x=w41, y=w43) -> (x .or. y?=w42:bool)
      }
      frame True {
      }
    }
    n795 = Unbundle By Name(w31) -> ("Current"=→"current":dbl, "Serial No"=→"Device serial number":string, "Status"=→"Potentiostat Status":string)
    n796 = Or(x=w25, y=w36) -> (x .or. y?=w35:bool)
    n797 = case shown="False" w20 {
      tunnel: w7 -> [w85 w86]
      tunnel: [w85 w86] -> w21
      frame False {
      }
      frame True {
        n798 = disable-structure shown="Disabled" {
          disable-tunnel: [State."Exit" ("f") _] -> _
          frame Disabled {
            n799 = call "Display Message to User"() -> ()  [unwired: 10 in, 2 out]
          }
          frame Enabled {
          }
        }
      }
    }
  }
